vi "Competition.vi"() -> ()   [LabVIEW 2024]
uses:
  <vilib>/userDefined/High Color/IMAQdx.ctl
  System.Windows.Forms
  <vilib>/Instr/_visa.llb/VISA Set IO Buffer Mask.ctl
  <vilib>/Instr/_visa.llb/VISA Flush IO Buffer Mask.ctl
  e33ea129-5426-40bd-9da2-e127971607b1.vi
  <vilib>/Instr/_visa.llb/VISA Configure Serial Port (Instr).vi
  <vilib>/Python/Open Venv Python Session.vi
  <vilib>/Utility/file.llb/Read Delimited Spreadsheet (DBL).vi
  <vilib>/vision/driver/NI_Vision_Acquisition_Software.lvlib
panel:
  in  "RDDF":path=path "C:/Users/JungiHong/OneDrive/Hongik/HI-RACE/2026-01/ExperimentModules/GPSPathTracking/1_5_map/1_5_map hard.txt"
  out "WP_no.":i32=675
  out "Path_lat_arr":dbl[](array[numeric])=[250246.8301, 250246.6716, 250246.4873, 250246.296, 250246.122, 250245.9257, 250245.7732, 250245.5875, 250245.3989, 250245.2166, 250245.0276, 250244.8653, 250244.6749, 250244.5098, 250244.319, 250244.1293, 250243.9404, 250243.757, 250243.5653, 250243.3909, 250243.2171, 250243.0265, 250242.8469, 250242.6561, 250242.4779, 250242.2931, 250242.1112, 250241.9363, 250241.7611, 250241.5908]
  out "Path_long_arr":dbl[](array[numeric])=[3688223.612, 3688223.681, 3688223.731, 3688223.77, 3688223.796, 3688223.82, 3688223.842, 3688223.793, 3688223.791, 3688223.745, 3688223.702, 3688223.665, 3688223.63, 3688223.575, 3688223.538, 3688223.496, 3688223.445, 3688223.39, 3688223.345, 3688223.293, 3688223.242, 3688223.21, 3688223.151, 3688223.108, 3688223.058, 3688223.007, 3688222.954, 3688222.905, 3688222.836, 3688222.787]
  out "Path_Vel_arr":dbl[](array[numeric])=[126.3175841, 126.3175824, 126.3175804, 126.3175784, 126.3175765, 126.3175744, 126.3175727, 126.3175708, 126.3175687, 126.3175668, 126.3175648, 126.3175631, 126.317561, 126.3175593, 126.3175572, 126.3175552, 126.3175532, 126.3175512, 126.3175492, 126.3175473, 126.3175455, 126.3175434, 126.3175415, 126.3175395, 126.3175376, 126.3175356, 126.3175337, 126.3175318, 126.31753, 126.3175282]
  out "Path_Evt_arr":dbl[](array[numeric])=[33.30420584, 33.30420642, 33.30420683, 33.30420714, 33.30420733, 33.3042075, 33.30420766, 33.30420718, 33.30420712, 33.30420667, 33.30420623, 33.30420586, 33.3042055, 33.30420497, 33.30420459, 33.30420417, 33.30420367, 33.30420313, 33.30420267, 33.30420217, 33.30420167, 33.30420133, 33.30420076, 33.30420033, 33.30419983, 33.30419933, 33.30419882, 33.30419833, 33.30419768, 33.30419719]
  out "Evt":dbl
  in  "Map Refresh":bool
  out "X_lat_path_Full":dbl[](array[numeric])=[250204.6315, 250204.7847, 250204.9423, 250205.0812, 250205.2434, 250205.3871, 250205.5336, 250205.6795, 250205.8333, 250205.974, 250206.1254, 250206.2733, 250206.4155, 250206.5694, 250206.7606, 250206.9331, 250207.0915, 250207.2338, 250207.3801, 250207.5358, 250207.6911, 250207.8385, 250207.9859, 250208.1346, 250208.2889, 250208.4191, 250208.562, 250208.7088, 250208.8428, 250208.9854, 250209.1251, 250209.2579, 250209.3978, 250209.5384, 250209.6838, 250209.8317, 250209.9732, 250210.1069, 250210.2502, 250210.372, 250210.5044, 250210.6376, 250210.7611, 250210.9066, 250211.0503, 250211.1744, 250211.309, 250211.4462, 250211.5776, 250211.7104, 250211.8353, 250211.9552, 250212.0902, 250212.213, 250212.3298, 250212.4572, 250212.5757, 250212.6937, 250212.8209, 250212.9386, 250213.0558, 250213.1735, 250213.2937, 250213.4125, 250213.5502, 250213.6657, 250213.7946, 250213.9274, 250214.0472, 250214.1724, 250214.3017, 250214.4417, 250214.5753, 250214.7017, 250214.8378, 250214.9662, 250215.0894, 250215.2277, 250215.372, 250215.5023, 250215.6465, 250215.6465, 250215.7658, 250215.8914, 250216.017, 250216.142, 250216.2785, 250216.4267, 250216.5776, 250216.7312, 250216.8879, 250217.0506, 250217.2131, 250217.3799, 250217.5426, 250217.7046, 250217.8748, 250218.0423, 250218.2058, 250218.3739, 250218.5355, 250218.7031, 250218.8647, 250219.0346, 250219.1961, 250219.3482, 250219.5145, 250219.672, 250219.8212, 250219.9767, 250220.1301, 250220.2837, 250220.4332, 250220.5777, 250220.7226, 250220.8672, 250221.0139, 250221.1635, 250221.2913, 250221.4361, 250221.5854, 250221.7202, 250221.862, 250222.0043, 250222.1442, 250222.2947, 250222.4297, 250222.5803, 250222.7124, 250222.8553, 250222.9875, 250223.1252, 250223.2779, 250223.409, 250223.5472, 250223.6863, 250223.8257, 250223.9601, 250224.1026, 250224.2408, 250224.3821, 250224.528, 250224.675, 250224.8272, 250224.9781, 250225.124, 250225.2738, 250225.4183, 250225.5696, 250225.7148, 250225.8666, 250226.0158, 250226.1696, 250226.314, 250226.464, 250226.616, 250226.7669, 250226.8995, 250227.0551, 250227.2017, 250227.3491, 250227.4987, 250227.651, 250227.8032, 250227.9491, 250228.1012, 250228.2468, 250228.3977, 250228.5421, 250228.6906, 250228.8411, 250228.9881, 250229.1171, 250229.2733, 250229.4177, 250229.5665, 250229.7135, 250229.8553, 250229.9955, 250230.1399, 250230.2778, 250230.4184, 250230.5592, 250230.6982, 250230.8426, 250230.9741, 250231.1183, 250231.2583, 250231.3917, 250231.5316, 250231.664, 250231.809, 250231.9365, 250232.0794, 250232.2326, 250232.3781, 250232.5288, 250232.6849, 250232.849, 250233.0169, 250233.1898, 250233.3618, 250233.5347, 250233.7129, 250233.8854, 250234.0582, 250234.2271, 250234.392, 250234.5465, 250234.6882, 250234.8252, 250234.962, 250235.0951, 250235.2304, 250235.3491, 250235.4717, 250235.6036, 250235.7176, 250235.8287, 250235.9455, 250236.054, 250236.1492, 250236.2337, 250236.312, 250236.3794, 250236.4369, 250236.4842, 250236.5555, 250236.5952, 250236.6264, 250236.6586, 250236.6755, 250236.6895, 250236.6942, 250236.697, 250236.6851, 250236.6654, 250236.6292, 250236.5933, 250236.551, 250236.4843, 250236.4291, 250236.3642, 250236.3049, 250236.2381, 250236.1715, 250236.0948, 250236.0356, 250235.9406, 250235.8714, 250235.7898, 250235.7058, 250235.658, 250235.5758, 250235.4943, 250235.4193, 250235.3767, 250235.3402, 250235.2889, 250235.2668, 250235.2332, 250235.1891, 250235.1614, 250235.1565, 250235.1204, 250235.1167, 250235.133, 250235.1628, 250235.1974, 250235.2612, 250235.3531, 250235.4155, 250235.5356, 250235.6584, 250235.7924, 250235.9326, 250236.0835, 250236.1855, 250236.3061, 250236.46, 250236.5583, 250236.7204, 250236.8858, 250237.0619, 250237.2443, 250237.4126, 250237.579, 250237.7347, 250237.9052, 250238.0628, 250238.1948, 250238.3334, 250238.4969, 250238.6626, 250238.831, 250239.0118, 250239.1778, 250239.3373, 250239.5311, 250239.6876, 250239.8513, 250240.05, 250240.2334, 250240.4321, 250240.6256, 250240.816, 250240.9998, 250241.1899, 250241.3681, 250241.5524, 250241.7339, 250241.9189, 250242.1048, 250242.2826, 250242.4514, 250242.6353, 250242.8115, 250242.986, 250243.1671, 250243.3465, 250243.5187, 250243.6972, 250243.888, 250244.084, 250244.2833, 250244.4766, 250244.6711, 250244.8658, 250245.0556, 250245.2439, 250245.4299, 250245.6119, 250245.7785, 250245.9451, 250246.096, 250246.2496, 250246.3875, 250246.5144, 250246.631, 250246.7342, 250246.8204, 250246.907, 250247.0092, 250247.1016, 250247.193, 250247.2639, 250247.3441, 250247.421, 250247.4764, 250247.5347, 250247.5768, 250247.6199, 250247.652, 250247.665, 250247.6714, 250247.6666, 250247.6394, 250247.6096, 250247.5413, 250247.498, 250247.4546, 250247.3884, 250247.3334, 250247.2883, 250247.2288, 250247.1836, 250247.1639, 250247.1466, 250247.1079, 250247.1021, 250247.0827, 250247.0531, 250247.0114, 250247.0067, 250246.9862, 250246.9811, 250246.9938, 250247.0308, 250247.0702, 250247.135, 250247.2146, 250247.3014, 250247.4225, 250247.5588, 250247.6858, 250247.828, 250247.9565, 250248.126, 250248.2664, 250248.409, 250248.5611, 250248.7068, 250248.8531, 250249.0229, 250249.202, 250249.3857, 250249.5753, 250249.7637, 250249.959, 250250.1426, 250250.3367, 250250.5143, 250250.6887, 250250.882, 250251.0751, 250251.2683, 250251.4599, 250251.6407, 250251.8269, 250252.0222, 250252.215, 250252.3883, 250252.58, 250252.7757, 250252.9624, 250253.1529, 250253.3403, 250253.5294, 250253.7184, 250253.907, 250254.0796, 250254.2588, 250254.4147, 250254.5819, 250254.743, 250254.8895, 250255.0112, 250255.1568, 250255.2877, 250255.437, 250255.5889, 250255.7462, 250255.9147, 250256.0842, 250256.2597, 250256.4476, 250256.6251, 250256.814, 250257.0016, 250257.1907, 250257.383, 250257.5732, 250257.7644, 250257.9556, 250258.1438, 250258.3228, 250258.5095, 250258.6883, 250258.8678, 250259.0368, 250259.2086, 250259.3646, 250259.5205, 250259.6669, 250259.7981, 250259.9204, 250260.0341, 250260.1304, 250260.2154, 250260.2683, 250260.3212, 250260.3713, 250260.4074, 250260.4278, 250260.4483, 250260.4538, 250260.4584, 250260.4638, 250260.4531, 250260.4269, 250260.4025, 250260.3748, 250260.3569, 250260.3259, 250260.306, 250260.3019, 250260.2913, 250260.2964, 250260.3013, 250260.322, 250260.3442, 250260.3803, 250260.414, 250260.462, 250260.5251, 250260.6072, 250260.6942, 250260.7672, 250260.8711, 250260.9697, 250261.0724, 250261.1817, 250261.2963, 250261.3941, 250261.4821, 250261.569, 250261.6706, 250261.7652, 250261.857, 250261.9183, 250261.9427, 250261.9912, 250261.9961, 250262.0007, 250261.9756, 250261.9489, 250261.9099, 250261.8812, 250261.8445, 250261.7817, 250261.7129, 250261.6398, 250261.5329, 250261.4604, 250261.3434, 250261.24, 250261.1259, 250260.9928, 250260.8741, 250260.7678, 250260.6137, 250260.4623, 250260.2939, 250260.126, 250259.9411, 250259.7546, 250259.5669, 250259.4199, 250259.2239, 250259.0425, 250258.8499, 250258.6584, 250258.475, 250258.2939, 250258.1037, 250257.9137, 250257.7231, 250257.5553, 250257.3716, 250257.2069, 250257.0301, 250256.8666, 250256.6854, 250256.514, 250256.3482, 250256.1782, 250256.0288, 250255.8463, 250255.6842, 250255.5166, 250255.3463, 250255.1982, 250255.0421, 250254.892, 250254.7261, 250254.5713, 250254.4091, 250254.2573, 250254.0995, 250253.9355, 250253.7624, 250253.5867, 250253.3985, 250253.2139, 250253.0287, 250252.8354, 250252.6448, 250252.4492, 250252.2513, 250252.0571, 250251.8685, 250251.6866, 250251.5105, 250251.3443, 250251.1824, 250251.0309, 250250.8789, 250250.7367, 250250.5995, 250250.4539, 250250.3121, 250250.1719, 250250.0299, 250249.887, 250249.7463, 250249.6052, 250249.4649, 250249.331, 250249.1893, 250249.0528, 250248.9386, 250248.8243, 250248.7236, 250248.6306, 250248.529, 250248.4359, 250248.3517, 250248.2827, 250248.2037, 250248.1463, 250248.0957, 250248.0509, 250248.0219, 250248.0051, 250247.9945, 250247.9837, 250247.989, 250247.9941, 250247.9993, 250248.0044, 250248.0095, 250248.0145, 250248.0352, 250248.0557, 250248.0919, 250248.1148, 250248.1615, 250248.1868, 250248.2214, 250248.2728, 250248.3179, 250248.3416, 250248.3511, 250248.3839, 250248.4042, 250248.432, 250248.4459, 250248.4908, 250248.5037, 250248.5435, 250248.5875, 250248.6237, 250248.6436, 250248.6662, 250248.6992, 250248.705, 250248.7258, 250248.7267, 250248.7214, 250248.7308, 250248.744, 250248.7337, 250248.7226, 250248.6855, 250248.6674, 250248.5843, 250248.537, 250248.448, 250248.3765, 250248.2712, 250248.1941, 250248.1144, 250247.9992, 250247.891, 250247.7807, 250247.6307, 250247.5171, 250247.3602, 250247.1874, 250247.0166, 250246.8301, 250246.6716, 250246.4873, 250246.296, 250246.122, 250245.9257, 250245.7732, 250245.5875, 250245.3989, 250245.2166, 250245.0276, 250244.8653, 250244.6749, 250244.5098, 250244.319, 250244.1293, 250243.9404, 250243.757, 250243.5653, 250243.3909, 250243.2171, 250243.0265, 250242.8469, 250242.6561, 250242.4779, 250242.2931, 250242.1112, 250241.9363, 250241.7611, 250241.5908, 250241.4105, 250241.2326, 250241.0415, 250240.8823, 250240.7086, 250240.5237, 250240.3385, 250240.1546, 250239.9595, 250239.7651, 250239.5694, 250239.3713, 250239.1737, 250238.9795, 250238.7874, 250238.5977, 250238.4158, 250238.2247, 250238.0451, 250237.867, 250237.6942, 250237.5189, 250237.359, 250237.1898, 250237.0315, 250236.8728, 250236.7137, 250236.5718, 250236.437, 250236.2994, 250236.1879, 250236.0639, 250235.9389, 250235.83, 250235.7229, 250235.6297, 250235.5351, 250235.4494, 250235.3697, 250235.3065, 250235.2435, 250235.1994, 250235.1375, 250235.0894, 250235.041, 250235.0127, 250234.9717, 250234.9373, 250234.9195, 250234.8912, 250234.852, 250234.8256, 250234.8066, 250234.7894, 250234.7971, 250234.798, 250234.7875, 250234.8083, 250234.8039, 250234.8027, 250234.8079, 250234.813, 250234.8181, 250234.8119, 250234.8202, 250234.8152, 250234.8222, 250234.8216, 250234.7975, 250234.7903, 250234.7485, 250234.7087, 250234.6504, 250234.616, 250234.567, 250234.5014, 250234.4497, 250234.3789, 250234.3334, 250234.2602, 250234.1655, 250234.0706, 250233.9596, 250233.8482, 250233.6928, 250233.5374, 250233.4092, 250233.2698, 250233.1115, 250232.9573, 250232.785, 250232.598, 250232.4051, 250232.2295, 250232.0509, 250231.866, 250231.6857, 250231.4995, 250231.3134, 250231.1433, 250230.9457, 250230.7492, 250230.5768, 250230.3831, 250230.1894, 250229.9975, 250229.8111, 250229.6241, 250229.4384, 250229.2517, 250229.069, 250228.8781, 250228.6895, 250228.511, 250228.3291, 250228.1418, 250227.9599, 250227.7698, 250227.597, 250227.4079, 250227.2175, 250227.0293, 250226.8363, 250226.6397, 250226.4445, 250226.4445, 250226.3195, 250226.1946, 250226.0696, 250225.9221, 250225.7742, 250225.6168, 250225.47, 250225.3233, 250225.1765, 250225.0287, 250224.8822, 250224.7443, 250224.5996, 250224.4528, 250224.301, 250224.1558, 250224.0269, 250223.8866, 250223.7351, 250223.5855, 250223.4444, 250223.2886, 250223.148, 250223.0104, 250222.8695, 250222.7295, 250222.5838, 250222.4554, 250222.316, 250222.1912, 250222.056, 250221.9297, 250221.7922, 250221.6642, 250221.5466, 250221.3995, 250221.2768, 250221.1432, 250221.0095, 250220.8891, 250220.7597, 250220.6502, 250220.5287, 250220.4116, 250220.2851, 250220.1647, 250220.0444, 250219.9261, 250219.7966, 250219.6741, 250219.5628, 250219.4354, 250219.3182, 250219.1887, 250219.0582, 250218.9251, 250218.8036, 250218.679, 250218.5495, 250218.4169, 250218.2866, 250218.1513, 250218.0199, 250217.8896, 250217.7568, 250217.6185, 250217.4845, 250217.3551, 250217.2166, 250217.0853, 250216.9453, 250216.8055, 250216.6585, 250216.5131, 250216.3689, 250216.2118, 250216.0655, 250215.9129, 250215.7606, 250215.6071, 250215.4505, 250215.2942, 250215.1411, 250214.9841, 250214.842, 250214.6871, 250214.5483, 250214.3987, 250214.2557, 250214.1195, 250213.9747, 250213.8377, 250213.7044, 250213.5703, 250213.4445, 250213.3184, 250213.183, 250213.0559, 250212.9317, 250212.8112, 250212.6789, 250212.5512, 250212.4267, 250212.2918, 250212.1645, 250212.0429, 250211.9046, 250211.769, 250211.6308, 250211.492, 250211.3609, 250211.2259, 250211.0952, 250210.9578, 250210.8141, 250210.6818, 250210.5388, 250210.4096, 250210.2669, 250210.1265, 250209.986, 250209.8443, 250209.696, 250209.5582, 250209.4275, 250209.2882, 250209.1319, 250209.0284]
  out "vel. path":dbl[](array[numeric])=[126.317125, 126.3171267, 126.3171284, 126.3171299, 126.3171317, 126.3171333, 126.3171349, 126.3171365, 126.3171382, 126.3171397, 126.3171414, 126.317143, 126.3171446, 126.3171463, 126.3171483, 126.3171502, 126.317152, 126.3171535, 126.3171551, 126.3171568, 126.3171585, 126.3171601, 126.3171618, 126.3171634, 126.3171651, 126.3171665, 126.3171681, 126.3171697, 126.3171712, 126.3171728, 126.3171743, 126.3171758, 126.3171773, 126.3171788, 126.3171804, 126.3171821, 126.3171836, 126.3171851, 126.3171867, 126.317188, 126.3171895, 126.317191, 126.3171923, 126.3171939, 126.3171955, 126.3171969, 126.3171984, 126.3171999, 126.3172013, 126.3172028, 126.3172042, 126.3172055, 126.317207, 126.3172083, 126.3172096, 126.3172111, 126.3172124, 126.3172137, 126.3172151, 126.3172164, 126.3172177, 126.317219, 126.3172203, 126.3172217, 126.3172232, 126.3172245, 126.3172259, 126.3172273, 126.3172287, 126.3172301, 126.3172315, 126.317233, 126.3172345, 126.3172359, 126.3172374, 126.3172388, 126.3172402, 126.3172417, 126.3172433, 126.3172447, 126.3172463, 126.3172463, 126.3172476, 126.317249, 126.3172504, 126.3172518, 126.3172533, 126.3172549, 126.3172566, 126.3172583, 126.31726, 126.3172618, 126.3172635, 126.3172654, 126.3172671, 126.3172689, 126.3172708, 126.3172726, 126.3172744, 126.3172762, 126.317278, 126.3172798, 126.3172816, 126.3172834, 126.3172852, 126.3172868, 126.3172886, 126.3172904, 126.317292, 126.3172937, 126.3172954, 126.3172971, 126.3172987, 126.3173003, 126.3173019, 126.3173035, 126.3173051, 126.3173067, 126.3173081, 126.3173097, 126.3173114, 126.3173129, 126.3173144, 126.317316, 126.3173175, 126.3173192, 126.3173207, 126.3173223, 126.3173238, 126.3173253, 126.3173268, 126.3173283, 126.31733, 126.3173314, 126.317333, 126.3173345, 126.317336, 126.3173375, 126.3173391, 126.3173406, 126.3173421, 126.3173437, 126.3173454, 126.317347, 126.3173487, 126.3173503, 126.3173519, 126.3173535, 126.3173552, 126.3173568, 126.3173584, 126.3173601, 126.3173617, 126.3173633, 126.317365, 126.3173666, 126.3173683, 126.3173698, 126.3173715, 126.3173731, 126.3173747, 126.3173763, 126.317378, 126.3173797, 126.3173813, 126.3173829, 126.3173845, 126.3173862, 126.3173878, 126.3173894, 126.3173911, 126.3173927, 126.3173941, 126.3173958, 126.3173974, 126.317399, 126.3174006, 126.3174022, 126.3174037, 126.3174053, 126.3174068, 126.3174084, 126.3174099, 126.3174115, 126.3174131, 126.3174145, 126.3174161, 126.3174176, 126.3174191, 126.3174206, 126.3174221, 126.3174237, 126.3174251, 126.3174267, 126.3174284, 126.31743, 126.3174316, 126.3174333, 126.3174351, 126.3174369, 126.3174388, 126.3174407, 126.3174426, 126.3174445, 126.3174464, 126.3174483, 126.3174501, 126.3174519, 126.3174536, 126.3174552, 126.3174567, 126.3174582, 126.3174596, 126.3174611, 126.3174624, 126.3174638, 126.3174653, 126.3174665, 126.3174678, 126.3174691, 126.3174703, 126.3174713, 126.3174723, 126.3174732, 126.317474, 126.3174746, 126.3174752, 126.317476, 126.3174765, 126.3174769, 126.3174773, 126.3174775, 126.3174777, 126.3174778, 126.3174779, 126.3174778, 126.3174777, 126.3174773, 126.317477, 126.3174766, 126.3174759, 126.3174754, 126.3174748, 126.3174742, 126.3174735, 126.3174728, 126.3174721, 126.3174715, 126.3174705, 126.3174698, 126.317469, 126.3174681, 126.3174677, 126.3174668, 126.317466, 126.3174653, 126.3174648, 126.3174645, 126.317464, 126.3174638, 126.3174635, 126.3174631, 126.3174628, 126.3174628, 126.3174625, 126.3174625, 126.3174627, 126.3174631, 126.3174635, 126.3174643, 126.3174653, 126.317466, 126.3174673, 126.3174687, 126.3174702, 126.3174717, 126.3174734, 126.3174745, 126.3174758, 126.3174775, 126.31747849999999, 126.3174803, 126.3174821, 126.317484, 126.317486, 126.3174878, 126.3174896, 126.3174913, 126.3174932, 126.3174949, 126.3174963, 126.3174978, 126.3174996, 126.3175014, 126.3175032, 126.3175052, 126.317507, 126.3175087, 126.3175108, 126.3175125, 126.3175142, 126.3175164, 126.3175183, 126.3175205, 126.3175225, 126.3175246, 126.3175265, 126.3175286, 126.3175305, 126.3175324, 126.3175344, 126.3175363, 126.3175383, 126.3175402, 126.317542, 126.3175439, 126.3175458, 126.3175477, 126.3175496, 126.3175515, 126.3175533, 126.3175552, 126.3175573, 126.3175594, 126.3175615, 126.3175636, 126.3175657, 126.3175678, 126.3175698, 126.3175719, 126.3175739, 126.3175759, 126.3175777, 126.3175795, 126.3175811, 126.3175828, 126.3175843, 126.3175857, 126.317587, 126.3175882, 126.3175892, 126.3175901, 126.3175913, 126.3175923, 126.3175933, 126.3175942, 126.3175951, 126.3175959, 126.3175966, 126.3175973, 126.3175978, 126.3175983, 126.3175987, 126.3175989, 126.317599, 126.317599, 126.3175988, 126.3175985, 126.3175978, 126.3175974, 126.317597, 126.3175963, 126.3175958, 126.3175954, 126.3175948, 126.3175943, 126.3175942, 126.317594, 126.3175937, 126.3175937, 126.3175935, 126.3175932, 126.3175928, 126.3175928, 126.3175927, 126.3175927, 126.3175929, 126.3175933, 126.3175938, 126.3175945, 126.3175954, 126.3175964, 126.3175977, 126.3175992, 126.3176006, 126.3176022, 126.3176036, 126.3176055, 126.317607, 126.3176086, 126.3176102, 126.3176118, 126.3176134, 126.3176152, 126.3176172, 126.3176192, 126.3176212, 126.3176233, 126.3176254, 126.3176274, 126.3176294, 126.3176314, 126.3176333, 126.3176353, 126.3176374, 126.3176395, 126.3176416, 126.3176435, 126.3176455, 126.3176476, 126.3176497, 126.3176515, 126.3176536, 126.3176557, 126.3176577, 126.3176597, 126.3176617, 126.3176637, 126.3176657, 126.3176677, 126.3176696, 126.3176715, 126.3176731, 126.3176749, 126.3176766, 126.3176781, 126.3176794, 126.3176809, 126.3176823, 126.3176838, 126.3176854, 126.3176871, 126.3176889, 126.3176906, 126.3176925, 126.3176945, 126.3176964, 126.3176984, 126.3177004, 126.3177024, 126.3177044, 126.3177065, 126.3177085, 126.3177106, 126.3177126, 126.3177145, 126.3177164, 126.3177183, 126.3177202, 126.317722, 126.3177238, 126.3177255, 126.3177271, 126.3177287, 126.31773, 126.3177313, 126.3177325, 126.3177335, 126.3177343, 126.3177348, 126.3177353, 126.3177358, 126.3177362, 126.3177363, 126.3177365, 126.3177365, 126.3177365, 126.3177365, 126.3177363, 126.317736, 126.3177357, 126.3177353, 126.3177351, 126.3177347, 126.3177344, 126.3177343, 126.3177342, 126.3177342, 126.3177342, 126.3177343, 126.3177345, 126.3177349, 126.3177352, 126.3177356, 126.3177362, 126.3177371, 126.317738, 126.3177387, 126.3177398, 126.3177408, 126.3177418, 126.317743, 126.3177441, 126.3177452, 126.317746, 126.3177469, 126.317748, 126.3177489, 126.3177499, 126.3177505, 126.3177507, 126.3177512, 126.3177512, 126.3177512, 126.3177508, 126.3177505, 126.31775, 126.3177497, 126.3177492, 126.3177485, 126.3177477, 126.3177469, 126.3177457, 126.3177449, 126.3177436, 126.3177424, 126.3177412, 126.3177397, 126.3177384, 126.3177372, 126.3177355, 126.3177339, 126.317732, 126.3177302, 126.3177282, 126.3177262, 126.3177242, 126.3177226, 126.3177205, 126.3177186, 126.3177165, 126.3177145, 126.3177125, 126.3177106, 126.3177085, 126.3177065, 126.3177045, 126.3177027, 126.3177007, 126.317699, 126.3176971, 126.3176954, 126.3176934, 126.3176916, 126.3176899, 126.3176881, 126.3176865, 126.3176845, 126.3176828, 126.3176811, 126.3176793, 126.3176777, 126.317676, 126.3176745, 126.3176727, 126.3176711, 126.3176694, 126.3176678, 126.3176661, 126.3176644, 126.3176626, 126.3176607, 126.3176587, 126.3176567, 126.3176548, 126.3176527, 126.3176507, 126.3176486, 126.3176464, 126.3176444, 126.3176423, 126.3176403, 126.3176384, 126.3176366, 126.3176349, 126.3176332, 126.3176315, 126.31763, 126.3176285, 126.3176269, 126.3176253, 126.3176238, 126.3176222, 126.3176206, 126.3176191, 126.3176175, 126.317616, 126.3176145, 126.3176129, 126.3176114, 126.3176102, 126.3176089, 126.3176078, 126.3176067, 126.3176056, 126.3176045, 126.3176036, 126.3176028, 126.3176019, 126.3176012, 126.3176006, 126.3176001, 126.3175997, 126.3175995, 126.3175993, 126.3175992, 126.3175992, 126.3175992, 126.3175992, 126.3175992, 126.3175992, 126.3175992, 126.3175993, 126.3175995, 126.3175998, 126.3176, 126.3176005, 126.3176007, 126.317601, 126.3176015, 126.3176019, 126.3176022, 126.3176022, 126.3176025, 126.3176027, 126.3176029, 126.317603, 126.3176034, 126.3176035, 126.3176039, 126.3176043, 126.3176047, 126.3176048, 126.317605, 126.3176053, 126.3176053, 126.3176055, 126.3176055, 126.3176054, 126.3176054, 126.3176055, 126.3176053, 126.3176052, 126.3176047, 126.3176045, 126.3176035, 126.317603, 126.317602, 126.3176012, 126.3176, 126.3175991, 126.3175982, 126.3175969, 126.3175957, 126.3175945, 126.3175929, 126.3175916, 126.3175899, 126.317588, 126.3175862, 126.3175841, 126.3175824, 126.3175804, 126.3175784, 126.3175765, 126.3175744, 126.3175727, 126.3175708, 126.3175687, 126.3175668, 126.3175648, 126.3175631, 126.317561, 126.3175593, 126.3175572, 126.3175552, 126.3175532, 126.3175512, 126.3175492, 126.3175473, 126.3175455, 126.3175434, 126.3175415, 126.3175395, 126.3175376, 126.3175356, 126.3175337, 126.3175318, 126.31753, 126.3175282, 126.3175262, 126.3175243, 126.3175223, 126.3175206, 126.3175188, 126.3175168, 126.3175148, 126.3175129, 126.3175108, 126.3175087, 126.3175066, 126.3175045, 126.3175024, 126.3175003, 126.3174982, 126.3174961, 126.3174942, 126.3174921, 126.3174902, 126.3174882, 126.3174863, 126.3174844, 126.3174827, 126.3174809, 126.3174791, 126.3174774, 126.3174756, 126.3174741, 126.3174726, 126.3174711, 126.3174698, 126.3174685, 126.3174671, 126.3174659, 126.3174647, 126.3174636, 126.3174626, 126.3174616, 126.3174607, 126.31746, 126.3174592, 126.3174587, 126.317458, 126.3174574, 126.3174568, 126.3174565, 126.317456, 126.3174556, 126.3174553, 126.317455, 126.3174545, 126.3174542, 126.3174539, 126.3174537, 126.3174537, 126.3174537, 126.3174535, 126.3174537, 126.3174536, 126.3174535, 126.3174535, 126.3174535, 126.3174535, 126.3174534, 126.3174534, 126.3174533, 126.3174533, 126.3174533, 126.317453, 126.3174528, 126.3174523, 126.3174519, 126.3174512, 126.3174508, 126.3174502, 126.3174494, 126.3174488, 126.317448, 126.3174475, 126.3174467, 126.3174456, 126.3174445, 126.3174433, 126.3174421, 126.3174404, 126.3174387, 126.3174373, 126.3174358, 126.317434, 126.3174324, 126.3174305, 126.3174285, 126.3174264, 126.3174245, 126.3174226, 126.3174206, 126.3174187, 126.3174167, 126.3174147, 126.3174128, 126.3174107, 126.3174086, 126.3174068, 126.3174047, 126.3174026, 126.3174006, 126.3173986, 126.3173966, 126.3173946, 126.3173926, 126.3173907, 126.3173887, 126.3173867, 126.3173848, 126.3173828, 126.3173808, 126.3173789, 126.3173769, 126.317375, 126.317373, 126.317371, 126.317369, 126.3173669, 126.31736480000001, 126.3173627, 126.3173627, 126.3173614, 126.31736, 126.3173587, 126.3173571, 126.3173554, 126.3173537, 126.3173521, 126.3173505, 126.3173489, 126.3173473, 126.3173457, 126.3173441, 126.3173426, 126.3173409, 126.3173393, 126.3173377, 126.3173363, 126.3173347, 126.3173331, 126.3173314, 126.3173299, 126.3173282, 126.3173266, 126.3173251, 126.3173235, 126.317322, 126.3173204, 126.317319, 126.3173175, 126.3173161, 126.3173146, 126.3173132, 126.3173117, 126.3173103, 126.3173089, 126.3173073, 126.317306, 126.3173045, 126.317303, 126.3173017, 126.3173003, 126.317299, 126.3172977, 126.3172964, 126.317295, 126.3172937, 126.3172923, 126.317291, 126.3172896, 126.3172882, 126.317287, 126.3172856, 126.3172843, 126.3172829, 126.3172814, 126.31728, 126.3172786, 126.3172772, 126.3172758, 126.3172743, 126.3172729, 126.3172714, 126.31727, 126.3172685, 126.317267, 126.3172655, 126.317264, 126.3172626, 126.3172611, 126.3172596, 126.3172581, 126.3172566, 126.317255, 126.3172534, 126.3172518, 126.3172501, 126.3172485, 126.3172468, 126.3172451, 126.3172434, 126.3172417, 126.31724, 126.3172383, 126.3172366, 126.3172351, 126.3172334, 126.3172318, 126.3172302, 126.3172286, 126.3172271, 126.3172255, 126.317224, 126.3172225, 126.3172211, 126.3172197, 126.3172183, 126.3172168, 126.3172154, 126.317214, 126.3172127, 126.3172112, 126.3172098, 126.3172084, 126.3172069, 126.3172055, 126.3172042, 126.3172027, 126.3172012, 126.3171997, 126.3171981, 126.3171967, 126.3171952, 126.3171937, 126.3171922, 126.3171907, 126.3171892, 126.3171876, 126.3171862, 126.3171846, 126.3171831, 126.3171815, 126.31718, 126.3171783, 126.3171768, 126.3171754, 126.3171739, 126.3171721, 126.317171]
  out "Y_long_path_Full":dbl[](array[numeric])=[3688246.636, 3688246.509, 3688246.386, 3688246.252, 3688246.131, 3688245.999, 3688245.863, 3688245.725, 3688245.593, 3688245.45, 3688245.315, 3688245.179, 3688245.039, 3688244.911, 3688244.843, 3688244.735, 3688244.608, 3688244.485, 3688244.347, 3688244.225, 3688244.098, 3688243.962, 3688243.826, 3688243.702, 3688243.576, 3688243.428, 3688243.289, 3688243.152, 3688243.019, 3688242.881, 3688242.758, 3688242.611, 3688242.466, 3688242.324, 3688242.184, 3688242.046, 3688241.912, 3688241.761, 3688241.621, 3688241.464, 3688241.317, 3688241.168, 3688241.016, 3688240.878, 3688240.743, 3688240.587, 3688240.445, 3688240.302, 3688240.154, 3688240.007, 3688239.85, 3688239.697, 3688239.549, 3688239.391, 3688239.229, 3688239.078, 3688238.919, 3688238.759, 3688238.606, 3688238.449, 3688238.288, 3688238.132, 3688237.972, 3688237.812, 3688237.667, 3688237.509, 3688237.359, 3688237.212, 3688237.056, 3688236.903, 3688236.761, 3688236.618, 3688236.472, 3688236.318, 3688236.18, 3688236.04, 3688235.882, 3688235.736, 3688235.602, 3688235.455, 3688235.317, 3688235.317, 3688235.161, 3688235.009, 3688234.859, 3688234.707, 3688234.563, 3688234.431, 3688234.301, 3688234.177, 3688234.058, 3688233.945, 3688233.832, 3688233.726, 3688233.616, 3688233.504, 3688233.406, 3688233.302, 3688233.192, 3688233.09, 3688232.98, 3688232.875, 3688232.767, 3688232.663, 3688232.554, 3688232.429, 3688232.322, 3688232.207, 3688232.075, 3688231.951, 3688231.826, 3688231.702, 3688231.575, 3688231.444, 3688231.311, 3688231.182, 3688231.047, 3688230.919, 3688230.774, 3688230.641, 3688230.511, 3688230.367, 3688230.231, 3688230.094, 3688229.957, 3688229.829, 3688229.683, 3688229.557, 3688229.413, 3688229.278, 3688229.132, 3688228.991, 3688228.865, 3688228.717, 3688228.577, 3688228.436, 3688228.296, 3688228.16, 3688228.023, 3688227.884, 3688227.749, 3688227.618, 3688227.486, 3688227.365, 3688227.239, 3688227.103, 3688226.975, 3688226.839, 3688226.711, 3688226.574, 3688226.45, 3688226.318, 3688226.199, 3688226.063, 3688225.934, 3688225.812, 3688225.684, 3688225.54, 3688225.421, 3688225.29, 3688225.156, 3688225.028, 3688224.9, 3688224.772, 3688224.642, 3688224.516, 3688224.383, 3688224.257, 3688224.124, 3688223.994, 3688223.865, 3688223.735, 3688223.59, 3688223.474, 3688223.338, 3688223.207, 3688223.074, 3688222.936, 3688222.795, 3688222.659, 3688222.518, 3688222.382, 3688222.244, 3688222.105, 3688221.97, 3688221.825, 3688221.694, 3688221.554, 3688221.407, 3688221.266, 3688221.121, 3688220.986, 3688220.837, 3688220.7, 3688220.579, 3688220.446, 3688220.321, 3688220.2, 3688220.09, 3688219.984, 3688219.886, 3688219.791, 3688219.695, 3688219.609, 3688219.511, 3688219.412, 3688219.312, 3688219.202, 3688219.08, 3688218.943, 3688218.802, 3688218.658, 3688218.514, 3688218.373, 3688218.215, 3688218.06, 3688217.916, 3688217.752, 3688217.592, 3688217.434, 3688217.271, 3688217.096, 3688216.918, 3688216.738, 3688216.555, 3688216.364, 3688216.175, 3688215.99, 3688215.797, 3688215.603, 3688215.408, 3688215.212, 3688215.018, 3688214.825, 3688214.629, 3688214.435, 3688214.238, 3688214.045, 3688213.854, 3688213.659, 3688213.473, 3688213.282, 3688213.096, 3688212.911, 3688212.732, 3688212.553, 3688212.373, 3688212.187, 3688212.026, 3688211.845, 3688211.666, 3688211.498, 3688211.307, 3688211.137, 3688210.957, 3688210.774, 3688210.583, 3688210.455, 3688210.27, 3688210.079, 3688209.89, 3688209.707, 3688209.511, 3688209.32, 3688209.133, 3688208.944, 3688208.778, 3688208.603, 3688208.425, 3688208.24, 3688208.069, 3688207.923, 3688207.776, 3688207.638, 3688207.505, 3688207.376, 3688207.261, 3688207.163, 3688207.105, 3688206.993, 3688206.89, 3688206.843, 3688206.777, 3688206.715, 3688206.655, 3688206.559, 3688206.461, 3688206.366, 3688206.273, 3688206.184, 3688206.113, 3688205.99, 3688205.895, 3688205.827, 3688205.775, 3688205.706, 3688205.658, 3688205.603, 3688205.616, 3688205.607, 3688205.608, 3688205.602, 3688205.579, 3688205.574, 3688205.595, 3688205.626, 3688205.67, 3688205.702, 3688205.765, 3688205.832, 3688205.892, 3688205.924, 3688205.975, 3688206.044, 3688206.125, 3688206.183, 3688206.249, 3688206.333, 3688206.409, 3688206.446, 3688206.526, 3688206.566, 3688206.595, 3688206.609, 3688206.603, 3688206.58, 3688206.556, 3688206.533, 3688206.491, 3688206.441, 3688206.381, 3688206.31, 3688206.213, 3688206.118, 3688205.996, 3688205.876, 3688205.735, 3688205.585, 3688205.428, 3688205.261, 3688205.087, 3688204.913, 3688204.745, 3688204.572, 3688204.399, 3688204.217, 3688204.041, 3688203.86, 3688203.671, 3688203.482, 3688203.291, 3688203.097, 3688202.903, 3688202.706, 3688202.51, 3688202.313, 3688202.121, 3688201.928, 3688201.742, 3688201.55, 3688201.357, 3688201.175, 3688201.009, 3688200.831, 3688200.66, 3688200.469, 3688200.293, 3688200.102, 3688199.927, 3688199.75, 3688199.553, 3688199.364, 3688199.207, 3688199.015, 3688198.819, 3688198.62, 3688198.43, 3688198.239, 3688198.051, 3688197.866, 3688197.706, 3688197.53, 3688197.389, 3688197.254, 3688197.113, 3688197.004, 3688196.877, 3688196.777, 3688196.671, 3688196.564, 3688196.467, 3688196.356, 3688196.256, 3688196.178, 3688196.107, 3688196.03, 3688195.977, 3688195.933, 3688195.904, 3688195.84, 3688195.809, 3688195.77, 3688195.714, 3688195.686, 3688195.663, 3688195.635, 3688195.597, 3688195.593, 3688195.569, 3688195.582, 3688195.578, 3688195.592, 3688195.622, 3688195.638, 3688195.688, 3688195.721, 3688195.771, 3688195.83, 3688195.888, 3688195.924, 3688196.013, 3688196.097, 3688196.199, 3688196.297, 3688196.407, 3688196.538, 3688196.689, 3688196.822, 3688196.969, 3688197.098, 3688197.223, 3688197.336, 3688197.437, 3688197.537, 3688197.627, 3688197.689, 3688197.772, 3688197.835, 3688197.898, 3688197.962, 3688198.006, 3688198.066, 3688198.118, 3688198.16, 3688198.22, 3688198.3, 3688198.363, 3688198.445, 3688198.523, 3688198.622, 3688198.722, 3688198.834, 3688198.951, 3688199.084, 3688199.233, 3688199.389, 3688199.552, 3688199.724, 3688199.899, 3688200.09, 3688200.276, 3688200.466, 3688200.659, 3688200.855, 3688201.049, 3688201.243, 3688201.442, 3688201.641, 3688201.837, 3688202.031, 3688202.224, 3688202.419, 3688202.615, 3688202.809, 3688203.003, 3688203.2, 3688203.398, 3688203.596, 3688203.795, 3688203.99, 3688204.187, 3688204.382, 3688204.576, 3688204.768, 3688204.955, 3688205.134, 3688205.302, 3688205.48, 3688205.649, 3688205.819, 3688205.987, 3688206.153, 3688206.315, 3688206.475, 3688206.647, 3688206.821, 3688206.984, 3688207.155, 3688207.331, 3688207.516, 3688207.707, 3688207.883, 3688208.081, 3688208.28, 3688208.475, 3688208.668, 3688208.858, 3688209.044, 3688209.226, 3688209.406, 3688209.585, 3688209.736, 3688209.892, 3688210.061, 3688210.21, 3688210.376, 3688210.537, 3688210.657, 3688210.774, 3688210.911, 3688211.029, 3688211.149, 3688211.236, 3688211.32, 3688211.383, 3688211.44, 3688211.445, 3688211.43, 3688211.417, 3688211.403, 3688211.371, 3688211.339, 3688211.288, 3688211.266, 3688211.231, 3688211.192, 3688211.159, 3688211.09, 3688211.04, 3688210.987, 3688210.902, 3688210.837, 3688210.775, 3688210.694, 3688210.621, 3688210.559, 3688210.478, 3688210.405, 3688210.295, 3688210.196, 3688210.103, 3688209.986, 3688209.897, 3688209.77, 3688209.673, 3688209.572, 3688209.462, 3688209.359, 3688209.244, 3688209.133, 3688209.036, 3688208.949, 3688208.891, 3688208.817, 3688208.749, 3688208.713, 3688208.664, 3688208.65, 3688208.66, 3688208.683, 3688208.737, 3688208.812, 3688208.9, 3688209.001, 3688209.113, 3688209.24, 3688209.367, 3688209.505, 3688209.64, 3688209.773, 3688209.904, 3688210.04, 3688210.178, 3688210.315, 3688210.453, 3688210.59, 3688210.727, 3688210.871, 3688211.008, 3688211.148, 3688211.311, 3688211.471, 3688211.642, 3688211.815, 3688211.983, 3688212.159, 3688212.339, 3688212.521, 3688212.701, 3688212.891, 3688213.083, 3688213.276, 3688213.469, 3688213.666, 3688213.862, 3688214.057, 3688214.255, 3688214.453, 3688214.653, 3688214.853, 3688215.051, 3688215.25, 3688215.444, 3688215.641, 3688215.834, 3688216.03, 3688216.22, 3688216.415, 3688216.609, 3688216.798, 3688216.975, 3688217.146, 3688217.341, 3688217.523, 3688217.718, 3688217.904, 3688218.088, 3688218.264, 3688218.452, 3688218.624, 3688218.803, 3688218.991, 3688219.18, 3688219.365, 3688219.554, 3688219.748, 3688219.937, 3688220.115, 3688220.312, 3688220.462, 3688220.658, 3688220.856, 3688221.033, 3688221.218, 3688221.387, 3688221.55, 3688221.723, 3688221.888, 3688222.066, 3688222.206, 3688222.378, 3688222.54, 3688222.688, 3688222.84, 3688222.985, 3688223.105, 3688223.246, 3688223.363, 3688223.459, 3688223.551, 3688223.612, 3688223.681, 3688223.731, 3688223.77, 3688223.796, 3688223.82, 3688223.842, 3688223.793, 3688223.791, 3688223.745, 3688223.702, 3688223.665, 3688223.63, 3688223.575, 3688223.538, 3688223.496, 3688223.445, 3688223.39, 3688223.345, 3688223.293, 3688223.242, 3688223.21, 3688223.151, 3688223.108, 3688223.058, 3688223.007, 3688222.954, 3688222.905, 3688222.836, 3688222.787, 3688222.74, 3688222.683, 3688222.638, 3688222.586, 3688222.511, 3688222.478, 3688222.412, 3688222.359, 3688222.34, 3688222.314, 3688222.3, 3688222.305, 3688222.31, 3688222.337, 3688222.376, 3688222.424, 3688222.483, 3688222.527, 3688222.608, 3688222.689, 3688222.783, 3688222.873, 3688222.992, 3688223.093, 3688223.213, 3688223.334, 3688223.454, 3688223.591, 3688223.737, 3688223.876, 3688224.034, 3688224.188, 3688224.344, 3688224.508, 3688224.673, 3688224.847, 3688225.02, 3688225.2, 3688225.381, 3688225.567, 3688225.754, 3688225.947, 3688226.135, 3688226.326, 3688226.518, 3688226.714, 3688226.903, 3688227.091, 3688227.284, 3688227.478, 3688227.672, 3688227.866, 3688228.052, 3688228.244, 3688228.437, 3688228.601, 3688228.797, 3688228.994, 3688229.189, 3688229.387, 3688229.587, 3688229.785, 3688229.985, 3688230.183, 3688230.38, 3688230.566, 3688230.748, 3688230.94, 3688231.128, 3688231.318, 3688231.504, 3688231.693, 3688231.866, 3688232.053, 3688232.23, 3688232.388, 3688232.573, 3688232.725, 3688232.88, 3688233.054, 3688233.218, 3688233.39, 3688233.528, 3688233.686, 3688233.804, 3688233.914, 3688234.006, 3688234.079, 3688234.157, 3688234.233, 3688234.306, 3688234.361, 3688234.397, 3688234.42, 3688234.426, 3688234.413, 3688234.415, 3688234.412, 3688234.395, 3688234.411, 3688234.397, 3688234.384, 3688234.363, 3688234.325, 3688234.303, 3688234.255, 3688234.209, 3688234.17, 3688234.122, 3688234.08, 3688234.02, 3688233.976, 3688233.93, 3688233.866, 3688233.809, 3688233.757, 3688233.697, 3688233.665, 3688233.601, 3688233.564, 3688233.533, 3688233.503, 3688233.455, 3688233.435, 3688233.422, 3688233.422, 3688233.413, 3688233.405, 3688233.397, 3688233.525, 3688233.659, 3688233.778, 3688233.911, 3688234.043, 3688234.174, 3688234.307, 3688234.435, 3688234.569, 3688234.705, 3688234.84, 3688234.961, 3688235.097, 3688235.227, 3688235.365, 3688235.493, 3688235.623, 3688235.758, 3688235.877, 3688236.014, 3688236.159, 3688236.295, 3688236.435, 3688236.571, 3688236.724, 3688236.867, 3688237.018, 3688237.158, 3688237.308, 3688237.453, 3688237.606, 3688237.764, 3688237.899, 3688238.054, 3688238.201, 3688238.349, 3688238.502, 3688238.644, 3688238.795, 3688238.953, 3688239.112, 3688239.259, 3688239.41, 3688239.562, 3688239.702, 3688239.853, 3688240.006, 3688240.166, 3688240.313, 3688240.473, 3688240.61, 3688240.762, 3688240.907, 3688241.061, 3688241.213, 3688241.362, 3688241.508, 3688241.659, 3688241.804, 3688241.946, 3688242.094, 3688242.243, 3688242.387, 3688242.527, 3688242.67, 3688242.808, 3688242.951, 3688243.091, 3688243.229, 3688243.354, 3688243.482, 3688243.612, 3688243.732, 3688243.857, 3688243.981, 3688244.094, 3688244.219, 3688244.343, 3688244.466, 3688244.587, 3688244.708, 3688244.84, 3688244.965, 3688245.103, 3688245.229, 3688245.362, 3688245.503, 3688245.64, 3688245.78, 3688245.922, 3688246.064, 3688246.214, 3688246.361, 3688246.508, 3688246.655, 3688246.809, 3688246.962, 3688247.108, 3688247.256, 3688247.407, 3688247.548, 3688247.695, 3688247.846, 3688247.99, 3688248.13, 3688248.271, 3688248.412, 3688248.553, 3688248.699, 3688248.848, 3688248.992, 3688249.128, 3688249.276, 3688249.41, 3688249.556, 3688249.69, 3688249.832, 3688249.967, 3688250.104, 3688250.232, 3688250.375, 3688250.521, 3688250.658, 3688250.777, 3688250.901]
  out "Evt.Arr":dbl[](array[numeric])=[33.3044035, 33.3044024, 33.30440132, 33.30440015, 33.3043991, 33.30439794, 33.30439675, 33.30439554, 33.30439439, 33.30439313, 33.30439195, 33.30439076, 33.30438953, 33.30438841, 33.30438784, 33.30438692, 33.3043858, 33.30438473, 33.30438352, 33.30438245, 33.30438134, 33.30438015, 33.30437896, 33.30437788, 33.30437678, 33.30437548, 33.30437425, 33.30437306, 33.30437189, 33.30437068, 33.3043696, 33.30436831, 33.30436703, 33.30436578, 33.30436456, 33.30436336, 33.30436217, 33.30436085, 33.30435962, 33.30435823, 33.30435694, 33.30435563, 33.30435428, 33.30435308, 33.30435189, 33.30435052, 33.30434926, 33.30434801, 33.30434672, 33.30434541, 33.30434403, 33.30434268, 33.30434137, 33.30433998, 33.30433855, 33.30433722, 33.30433581, 33.3043344, 33.30433306, 33.30433166, 33.30433024, 33.30432886, 33.30432745, 33.30432603, 33.30432476, 33.30432336, 33.30432204, 33.30432075, 33.30431937, 33.30431801, 33.30431677, 33.30431551, 33.30431422, 33.30431287, 33.30431166, 33.30431043, 33.30430903, 33.30430775, 33.30430658, 33.30430528, 33.30430407, 33.30430407, 33.30430269, 33.30430135, 33.30430003, 33.30429869, 33.30429743, 33.30429627, 33.30429513, 33.30429405, 33.30429302, 33.30429204, 33.30429106, 33.30429014, 33.30428918, 33.30428821, 33.30428737, 33.30428647, 33.30428552, 33.30428464, 33.30428368, 33.30428278, 33.30428184, 33.30428095, 33.30428, 33.30427891, 33.30427798, 33.30427698, 33.30427583, 33.30427475, 33.30427366, 33.30427257, 33.30427147, 33.30427032, 33.30426916, 33.30426802, 33.30426685, 33.30426572, 33.30426445, 33.30426329, 33.30426215, 33.30426088, 33.30425969, 33.30425848, 33.30425728, 33.30425617, 33.30425488, 33.30425379, 33.30425252, 33.30425133, 33.30425005, 33.30424881, 33.30424771, 33.3042464, 33.30424517, 33.30424394, 33.30424271, 33.30424152, 33.30424032, 33.30423909, 33.30423791, 33.30423676, 33.30423561, 33.30423456, 33.30423346, 33.30423226, 33.30423114, 33.30422995, 33.30422883, 33.30422763, 33.30422655, 33.3042254, 33.30422436, 33.30422317, 33.30422204, 33.30422098, 33.30421986, 33.30421859, 33.30421756, 33.30421641, 33.30421523, 33.30421412, 33.304213, 33.30421188, 33.30421074, 33.30420964, 33.30420848, 33.30420738, 33.30420621, 33.30420507, 33.30420395, 33.30420281, 33.30420153, 33.30420052, 33.30419933, 33.30419819, 33.30419702, 33.30419581, 33.30419457, 33.30419338, 33.30419214, 33.30419095, 33.30418974, 33.30418852, 33.30418734, 33.30418606, 33.30418491, 33.30418369, 33.3041824, 33.30418115, 33.30417988, 33.30417869, 33.30417738, 33.30417618, 33.30417512, 33.30417397, 33.30417287, 33.30417182, 33.30417087, 33.30416994, 33.3041691, 33.30416829, 33.30416747, 33.30416673, 33.30416589, 33.30416503, 33.30416417, 33.30416322, 33.30416216, 33.30416095, 33.30415971, 33.30415845, 33.30415719, 33.30415595, 33.30415455, 33.30415318, 33.30415192, 33.30415047, 33.30414905, 33.30414765, 33.30414621, 33.30414465, 33.30414307, 33.30414146, 33.30413983, 33.30413813, 33.30413643, 33.30413478, 33.30413306, 33.30413131, 33.30412956, 33.3041278, 33.30412605, 33.30412432, 33.30412256, 33.3041208, 33.30411902, 33.30411728, 33.30411554, 33.30411378, 33.30411208, 33.30411036, 33.30410866, 33.30410698, 33.30410535, 33.30410372, 33.30410208, 33.3041004, 33.30409893, 33.30409728, 33.30409564, 33.30409411, 33.30409238, 33.30409083, 33.30408919, 33.30408752, 33.30408579, 33.30408463, 33.30408295, 33.30408123, 33.30407952, 33.30407785, 33.30407608, 33.30407436, 33.30407267, 33.30407097, 33.30406947, 33.3040679, 33.3040663, 33.30406466, 33.30406313, 33.30406183, 33.30406054, 33.30405932, 33.30405816, 33.30405703, 33.30405602, 33.30405517, 33.30405467, 33.3040537, 33.3040528, 33.3040524, 33.30405185, 33.30405133, 33.30405083, 33.30405001, 33.30404917, 33.30404834, 33.30404755, 33.30404678, 33.30404617, 33.3040451, 33.30404427, 33.3040437, 33.30404327, 33.30404269, 33.3040423, 33.30404184, 33.304042, 33.30404195, 33.304042, 33.304042, 33.30404183, 33.30404183, 33.30404207, 33.30404239, 33.30404283, 33.30404317, 33.30404377, 33.30404442, 33.304045, 33.30404533, 33.30404583, 33.3040465, 33.30404726, 33.30404783, 33.30404846, 33.30404926, 33.30404999, 33.30405036, 33.30405112, 33.30405153, 33.30405183, 33.304052, 33.304052, 33.30405183, 33.30405167, 33.3040515, 33.30405117, 33.30405075, 33.30405026, 33.30404967, 33.30404883, 33.30404801, 33.30404694, 33.3040459, 33.30404467, 33.30404334, 33.30404195, 33.30404048, 33.30403893, 33.30403738, 33.30403588, 33.30403435, 33.30403281, 33.30403119, 33.30402962, 33.30402801, 33.30402632, 33.30402463, 33.30402292, 33.30402118, 33.30401944, 33.30401767, 33.3040159, 33.30401413, 33.30401239, 33.30401065, 33.30400895, 33.30400721, 33.30400546, 33.30400381, 33.3040023, 33.30400069, 33.30399913, 33.3039974, 33.30399581, 33.30399409, 33.3039925, 33.3039909, 33.30398913, 33.30398742, 33.30398599, 33.30398426, 33.30398249, 33.30398069, 33.30397899, 33.30397727, 33.30397559, 33.30397394, 33.30397251, 33.30397095, 33.30396971, 33.30396852, 33.30396728, 33.30396633, 33.30396522, 33.30396436, 33.30396343, 33.3039625, 33.30396166, 33.3039607, 33.30395983, 33.30395917, 33.30395857, 33.30395791, 33.30395748, 33.30395713, 33.30395691, 33.30395638, 33.30395615, 33.30395583, 33.30395537, 33.30395517, 33.303955, 33.30395479, 33.3039545, 33.3039545, 33.30395433, 33.30395449, 33.3039545, 33.30395467, 33.30395498, 33.30395517, 33.30395567, 33.303956, 33.3039565, 33.30395707, 33.30395764, 33.30395801, 33.30395885, 33.30395965, 33.3039606, 33.30396152, 33.30396255, 33.30396377, 33.30396516, 33.30396639, 33.30396774, 33.30396894, 33.3039701, 33.30397116, 33.30397211, 33.30397305, 33.3039739, 33.3039745, 33.30397529, 33.3039759, 33.30397652, 33.30397713, 33.30397757, 33.30397816, 33.30397867, 33.3039791, 33.30397968, 33.30398044, 33.30398105, 33.30398183, 33.30398257, 33.30398351, 33.30398444, 33.30398549, 33.30398658, 33.30398782, 33.30398919, 33.30399063, 33.30399212, 33.30399369, 33.30399528, 33.30399702, 33.3039987, 33.30400043, 33.30400218, 33.30400395, 33.3040057, 33.30400745, 33.30400925, 33.30401104, 33.30401281, 33.30401455, 33.30401628, 33.30401802, 33.30401979, 33.30402153, 33.30402328, 33.30402505, 33.30402683, 33.30402862, 33.30403041, 33.30403217, 33.30403395, 33.30403572, 33.30403748, 33.30403921, 33.30404092, 33.30404255, 33.30404408, 33.3040457, 33.30404725, 33.3040488, 33.30405033, 33.30405186, 33.30405334, 33.30405481, 33.30405638, 33.30405796, 33.30405946, 33.30406102, 33.30406263, 33.30406431, 33.30406604, 33.30406763, 33.30406942, 33.30407121, 33.30407296, 33.3040747, 33.3040764, 33.30407807, 33.3040797, 33.3040813, 33.3040829, 33.30408425, 33.30408563, 33.30408714, 33.30408845, 33.30408992, 33.30409134, 33.3040924, 33.30409342, 33.30409464, 33.30409566, 33.3040967, 33.30409745, 33.30409817, 33.30409869, 33.30409917, 33.30409917, 33.304099, 33.30409883, 33.30409867, 33.30409833, 33.304098, 33.3040975, 33.30409725, 33.3040969, 33.3040965, 33.30409617, 33.3040955, 33.304095, 33.30409449, 33.30409369, 33.30409306, 33.30409246, 33.30409169, 33.304091, 33.30409039, 33.30408964, 33.30408894, 33.3040879, 33.30408698, 33.30408609, 33.30408501, 33.30408417, 33.30408299, 33.30408207, 33.30408113, 33.30408011, 33.30407914, 33.30407806, 33.30407703, 33.30407611, 33.30407529, 33.30407472, 33.30407402, 33.30407336, 33.30407299, 33.3040725, 33.30407233, 33.30407238, 33.30407254, 33.30407298, 33.30407362, 33.30407437, 33.30407524, 33.30407621, 33.30407732, 33.30407842, 33.30407964, 33.30408083, 33.30408199, 33.30408313, 33.30408433, 33.30408554, 33.30408674, 33.30408795, 33.30408915, 33.30409035, 33.30409162, 33.30409282, 33.30409406, 33.3040955, 33.30409691, 33.30409843, 33.30409996, 33.30410145, 33.30410302, 33.30410462, 33.30410625, 33.30410785, 33.30410955, 33.30411127, 33.30411299, 33.30411473, 33.3041165, 33.30411826, 33.30412002, 33.3041218, 33.30412359, 33.30412539, 33.30412719, 33.30412898, 33.30413077, 33.30413253, 33.30413431, 33.30413605, 33.30413782, 33.30413955, 33.30414131, 33.30414306, 33.30414477, 33.30414638, 33.30414793, 33.30414969, 33.30415133, 33.3041531, 33.30415478, 33.30415644, 33.30415803, 33.30415973, 33.30416129, 33.30416291, 33.30416462, 33.30416633, 33.304168, 33.30416971, 33.30417146, 33.30417317, 33.30417477, 33.30417655, 33.3041779, 33.30417967, 33.30418145, 33.30418304, 33.3041847, 33.30418622, 33.30418767, 33.30418921, 33.30419068, 33.30419227, 33.3041935, 33.30419503, 33.30419648, 33.30419779, 33.30419913, 33.30420041, 33.30420146, 33.3042027, 33.30420372, 33.30420454, 33.30420533, 33.30420584, 33.30420642, 33.30420683, 33.30420714, 33.30420733, 33.3042075, 33.30420766, 33.30420718, 33.30420712, 33.30420667, 33.30420623, 33.30420586, 33.3042055, 33.30420497, 33.30420459, 33.30420417, 33.30420367, 33.30420313, 33.30420267, 33.30420217, 33.30420167, 33.30420133, 33.30420076, 33.30420033, 33.30419983, 33.30419933, 33.30419882, 33.30419833, 33.30419768, 33.30419719, 33.30419672, 33.30419617, 33.30419572, 33.30419522, 33.3041945, 33.30419416, 33.30419352, 33.304193, 33.30419279, 33.3041925, 33.30419233, 33.30419233, 33.30419233, 33.30419253, 33.30419283, 33.30419322, 33.30419371, 33.30419407, 33.30419475, 33.30419544, 33.30419625, 33.30419702, 33.30419805, 33.30419893, 33.30419998, 33.30420102, 33.30420207, 33.30420327, 33.30420455, 33.30420578, 33.30420717, 33.30420853, 33.3042099, 33.30421136, 33.30421282, 33.30421437, 33.3042159, 33.30421751, 33.30421912, 33.30422079, 33.30422245, 33.30422418, 33.30422586, 33.30422757, 33.30422929, 33.30423105, 33.30423274, 33.30423443, 33.30423617, 33.3042379, 33.30423964, 33.30424139, 33.30424306, 33.30424479, 33.30424652, 33.304248, 33.30424976, 33.30425154, 33.3042533, 33.30425509, 33.30425689, 33.30425867, 33.30426047, 33.30426226, 33.30426403, 33.30426571, 33.30426735, 33.30426908, 33.30427076, 33.30427248, 33.30427415, 33.30427584, 33.30427738, 33.30427906, 33.30428065, 33.30428205, 33.3042837, 33.30428506, 33.30428645, 33.304288, 33.30428946, 33.30429098, 33.3042922, 33.3042936, 33.30429462, 33.30429558, 33.30429638, 33.304297, 33.30429767, 33.30429832, 33.30429893, 33.30429939, 33.30429967, 33.30429983, 33.30429985, 33.30429968, 33.30429967, 33.3042996, 33.3042994, 33.3042995, 33.30429933, 33.30429917, 33.30429894, 33.30429855, 33.30429831, 33.30429783, 33.30429737, 33.30429697, 33.3042965, 33.30429608, 33.3042955, 33.30429506, 33.3042946, 33.30429398, 33.30429343, 33.30429291, 33.30429233, 33.304292, 33.30429138, 33.304291, 33.30429068, 33.30429037, 33.30428989, 33.30428967, 33.3042895, 33.3042895, 33.3042894, 33.30428929, 33.30428919, 33.3042903, 33.30429148, 33.30429252, 33.30429368, 33.30429483, 33.30429598, 33.30429714, 33.30429826, 33.30429944, 33.30430063, 33.30430181, 33.30430287, 33.30430407, 33.3043052, 33.30430642, 33.30430753, 33.30430867, 33.30430985, 33.30431089, 33.3043121, 33.30431337, 33.30431456, 33.30431579, 33.30431698, 33.30431833, 33.30431958, 33.30432092, 33.30432214, 33.30432347, 33.30432474, 33.30432609, 33.30432748, 33.30432867, 33.30433003, 33.30433133, 33.30433263, 33.30433399, 33.30433523, 33.30433657, 33.30433797, 33.30433937, 33.30434067, 33.304342, 33.30434334, 33.30434457, 33.30434591, 33.30434725, 33.30434867, 33.30434997, 33.30435138, 33.30435259, 33.30435392, 33.3043552, 33.30435656, 33.3043579, 33.30435921, 33.3043605, 33.30436182, 33.3043631, 33.30436435, 33.30436565, 33.30436696, 33.30436823, 33.30436946, 33.30437072, 33.30437193, 33.30437319, 33.30437442, 33.30437563, 33.30437672, 33.30437784, 33.30437898, 33.30438002, 33.30438112, 33.3043822, 33.30438318, 33.30438427, 33.30438535, 33.30438643, 33.30438748, 33.30438854, 33.30438969, 33.30439078, 33.30439199, 33.30439309, 33.30439426, 33.30439549, 33.3043967, 33.30439793, 33.30439917, 33.30440042, 33.30440174, 33.30440304, 33.30440434, 33.30440563, 33.30440699, 33.30440833, 33.30440962, 33.30441093, 33.30441225, 33.30441349, 33.30441479, 33.30441613, 33.30441739, 33.30441862, 33.30441985, 33.3044211, 33.30442234, 33.30442362, 33.30442493, 33.3044262, 33.30442739, 33.30442869, 33.30442987, 33.30443116, 33.30443233, 33.30443357, 33.30443475, 33.30443596, 33.30443707, 33.30443833, 33.30443962, 33.30444082, 33.30444186, 33.30444294]
  out "GPS":T1(graph)=[{"y_long_path"=[250243.79385612707], "x_lat_path"=[3688223.5281783747]}, {"y_long_path"=[250243.757], "x_lat_path"=[3688223.39]}, {"y_long_path"=array[944 elements], "x_lat_path"=array[944 elements]}, {"y_long_path"=[250246.8301, 250246.6716, 250246.4873, 250246.296, 250246.122, 250245.9257, 250245.7732, 250245.5875, 250245.3989, 250245.2166, 250245.0276, 250244.8653, 250244.6749, 250244.5098, 250244.319, 250244.1293, 250243.9404, 250243.757, 250243.5653, 250243.3909, 250243.2171, 250243.0265, 250242.8469, 250242.6561, 250242.4779, 250242.2931, 250242.1112, 250241.9363, 250241.7611, 250241.5908], "x_lat_path"=[3688223.612, 3688223.681, 3688223.731, 3688223.77, 3688223.796, 3688223.82, 3688223.842, 3688223.793, 3688223.791, 3688223.745, 3688223.702, 3688223.665, 3688223.63, 3688223.575, 3688223.538, 3688223.496, 3688223.445, 3688223.39, 3688223.345, 3688223.293, 3688223.242, 3688223.21, 3688223.151, 3688223.108, 3688223.058, 3688223.007, 3688222.954, 3688222.905, 3688222.836, 3688222.787]}]
  out "CTE":dbl=-0.11220359033506931
  in  "K_GPS":dbl=1.0 format="%#_13g"
  out "Tracking_Err(m)":dbl=4862130.802033398
  out "RDDF_Velocity":dbl=126.317125
  in  "Ld(m)":dbl=5.0 format="%#_13g"
  out "GPS_Steer_CMD(Deg)":dbl=2.9943056426975447
  in  "Steer Selector":enum32{"Stanley Method", "Pure Pursuit"}(radio)
  out "xi":dbl=250243.3909
  out "yi":dbl=3688223.293
  out "True_Heading(deg)":dbl format="%#_15g"
  out "UTM X(E) INS":dbl format="%#_13g"
  out "UTM Y(N) INS":dbl format="%#_13g"
  out "GPS_Speed(kph)":dbl format="%#_g kph"
  out "GPS Buffer Read":string
  out "Latitude(deg)":dbl
  out "Logitude(deg)":dbl
  out "Altitude(m)":dbl
  in  "COM7":refnum<visa-resource-name>="COM3" caption="GPS_Com."
  out "CV Loop Time":u32=19558436
  out "Lane_Steer":dbl=3.1742774367668782
  in  "K_Vision":dbl=1.0
  in  "v(Velocity)m/s":dbl=1.0
  out "inference time":string="Total: 586.3ms"
  in  "Binary_image":refnum<k24>(container)
  in  "Current_image":refnum<k24>(container)
  in  "min_area":u32=4
  in  "min_span":u32=4
  in  "max_rmse":u32=1000
  in  "kernel_size":u32=2
  in  "File Path":path=path "C:/Users/JungiHong/OneDrive/Hongik/HI-RACE/2026-01/platform_1_5/ExperimentModules/LaneTracking/forTrainImages/frame_014.jpg"
  in  "UseVideo":bool
  out "Image_String":string
  in  "Image Quality":u32=500
  in  "Cam No.":T2="cam3"
  out "Img_to_Str_Err":errorcluster
  in  "HENES":refnum<visa-resource-name>="COM7"
  out "E-STOP":bool
  out "Remote_M/A":bool
  out "Steer_Feed":dbl=-0.22
  out "Alive_PCU":u8(slide)=29 scale=0.0..254.0
  out "Gear_Feed":u8=1
  out "Speed_Feed(RPM)":dbl format="%#_g rpm"
  out "HENES Buffer Read":string
  out "Speed_Feed(m/s)":dbl
  in  "HLV_A/M":bool=TRUE
  in  "HLV_E-stop":bool
  out "HENES Buffer Write":string
  in  "Input_Spd(cmd)":dbl
  in  "GoBack":bool
  in  "InputSteer(cmd)":dbl
  in  "HLV_Gear":u8=2
  out "PointCloud":T3(graph)=[{"appended array"=[700.0, 700.0, 3500.0, 3500.0, -3500.0, -3500.0, -700.0, -700.0, 700.0], "appended array"=[800.0, -800.0, -800.0, 5200.0, 5200.0, -800.0, -800.0, 800.0, 800.0]}, {"appended array"=[-560.0], "appended array"=[0.0]}, {"appended array"=[-450.0, -450.0, -800.0, -800.0, 0.0, 0.0, -450.0], "appended array"=[100.0, -300.0, -300.0, 1200.0, 1200.0, 100.0, 100.0]}, {"appended array"=[], "appended array"=[]}, {"appended array"=[450.0, 450.0, 800.0, 800.0, 0.0, 0.0, 450.0], "appended array"=[100.0, -300.0, -300.0, 1200.0, 1200.0, 100.0, 100.0]}, {"appended array"=[-1100.0, -1100.0, -1120.0, -1120.0, -1140.0, -1140.0, -1140.0, -1160.0, -1160.0, -1160.0, -1180.0, -1180.0, -1180.0, -1200.0, -1200.0, -1200.0, -1220.0, -1220.0, -1220.0, -1220.0, -1240.0, -1260.0, -1260.0, -1260.0, -1280.0, -1280.0, -1280.0, -1280.0, -1300.0, -1300.0, -1300.0, -1320.0, -1320.0, -1320.0, -1340.0, -1340.0, -1340.0, -1360.0, -1360.0, -1360.0, -1380.0, -1380.0, -1380.0, -1400.0, -1400.0, -1400.0, -1420.0, -1420.0, -1420.0, -1440.0, -1440.0, -1440.0, -1460.0, -1460.0, -1460.0, -1480.0, -1480.0, -1480.0, -1500.0, -1500.0, -1500.0, -1500.0, -1520.0, -1520.0, -1520.0, -1540.0, -1540.0, -1540.0, -1560.0, -1560.0, -1560.0, -1580.0, -1580.0, -1580.0, -1600.0, -1600.0, -1600.0, -1620.0, -1620.0, -1620.0, -1640.0, -1640.0, -1660.0, -1660.0, -1680.0, -1680.0, -1680.0, -1700.0, -1700.0, -1720.0, -1720.0, -1720.0, -1740.0, -1740.0, -1760.0, -1760.0, -1760.0, -1780.0, -1780.0, -1800.0, -1800.0, -1820.0, -1820.0, -1840.0, -1840.0, -1860.0, -1860.0, -1880.0, -1880.0, -1900.0, -1920.0, -1920.0, -1940.0, -1960.0, -1980.0, -2000.0, -2020.0, -2040.0, -2040.0, -2060.0, -2060.0, -2100.0, -2120.0, -2120.0, -2120.0, -2140.0, -2160.0, -2180.0, -2200.0, -2220.0, -2240.0, -2260.0, -2280.0, -2300.0, -2320.0, -2360.0, -2380.0, -2400.0, -2440.0, -2460.0, -2480.0, -2520.0, -2520.0, -2540.0, -2980.0, -2960.0, -2960.0, -2940.0, 1180.0, 1200.0, 1220.0, 1220.0, 1240.0, 1260.0, 1260.0, 1280.0, 1380.0, 1380.0, 1380.0, 1400.0, 1400.0, 1420.0, 1420.0, 1440.0, 1460.0, 3460.0, 3460.0, 3460.0, 3460.0, 3480.0, 3480.0, 3500.0, -1646.388888888889, -2960.0, 1232.5, 1408.888888888889, 3471.4285714285716, 1252.0987654320988, 1271.6975308641975, 1291.2962962962963, 1310.8950617283951, 1330.4938271604938, 1350.0925925925926, 1369.6913580246915, 1389.29012345679], "appended array"=[40.0, 60.0, 60.0, 80.0, 80.0, 100.0, 120.0, 120.0, 140.0, 160.0, 180.0, 200.0, 220.0, 220.0, 240.0, 260.0, 260.0, 280.0, 300.0, 320.0, 340.0, 360.0, 380.0, 400.0, 400.0, 420.0, 440.0, 460.0, 460.0, 480.0, 500.0, 520.0, 540.0, 560.0, 560.0, 580.0, 600.0, 620.0, 640.0, 660.0, 660.0, 680.0, 700.0, 700.0, 720.0, 740.0, 740.0, 760.0, 780.0, 780.0, 800.0, 820.0, 840.0, 860.0, 880.0, 880.0, 900.0, 920.0, 920.0, 940.0, 960.0, 980.0, 980.0, 1000.0, 1020.0, 1020.0, 1040.0, 1060.0, 1080.0, 1100.0, 1120.0, 1120.0, 1140.0, 1160.0, 1160.0, 1180.0, 1200.0, 1220.0, 1240.0, 1260.0, 1280.0, 1300.0, 1320.0, 1340.0, 1360.0, 1380.0, 1400.0, 1420.0, 1440.0, 1460.0, 1480.0, 1500.0, 1520.0, 1540.0, 1560.0, 1580.0, 1600.0, 1620.0, 1640.0, 1660.0, 1680.0, 1700.0, 1720.0, 1740.0, 1780.0, 1800.0, 1820.0, 1840.0, 1860.0, 1920.0, 1940.0, 1980.0, 2020.0, 2080.0, 2120.0, 2160.0, 2180.0, 2220.0, 2240.0, 2280.0, 2320.0, 2360.0, 2400.0, 2420.0, 2460.0, 2500.0, 2540.0, 2580.0, 2620.0, 2680.0, 2720.0, 2780.0, 2820.0, 2880.0, 2920.0, 2980.0, 3020.0, 3080.0, 3160.0, 3220.0, 3280.0, 3340.0, 3380.0, 3440.0, 4340.0, 4360.0, 4380.0, 4420.0, 2560.0, 2580.0, 2560.0, 2540.0, 2540.0, 2540.0, 2520.0, 2520.0, 1720.0, 1700.0, 1680.0, 1680.0, 1660.0, 1660.0, 1640.0, 1660.0, 1660.0, 1800.0, 1780.0, 1760.0, 1740.0, 1720.0, 1700.0, 1700.0, 1304.1666666666667, 4375.0, 2545.0, 1673.3333333333333, 1742.857142857143, 2448.1481481481483, 2351.296296296296, 2254.4444444444443, 2157.5925925925926, 2060.740740740741, 1963.888888888889, 1867.037037037037, 1770.1851851851852]}, {"appended array"=[4.2861222383783204e-13, 0.0], "appended array"=[7000.0, 0.0]}, {"appended array"=[450.0, 450.0, -450.0, -450.0, 450.0], "appended array"=[100.0, 950.0, 950.0, 100.0, 100.0]}]
  in  "격자크기":dbl=20.0
  out "LidarLoop":u32=100
  in  "Ratio_Threshold":i32=4
  in  "min_samples":i32=2
  in  "eps":i32=100
  in  "Spacing":i32=100
  in  "Threshold":i32=2000
  in  "Looking Y":i32=5200
  in  "Looking X":i32=3500
  out "Anthena_Steer":i32
  out "NearSteer":dbl=71.42857142857143
  out "TooClose":bool=TRUE
  out "Clustering Loop":u32=100
  in  "LiDAR":refnum<visa-resource-name>="COM3"
  out "VEstop":bool
  in  "length":dbl=1300.0
  out "LiDAR Buffer Read":string
  out "Clustering Error":errorcluster
  out "GobackROI":cluster{i32[], i32[]}={[450, 450, -450, -450, 450], [100, 950, 950, 100, 100]}
  in  "Stop":bool
  out "TargetDerection":cluster{dbl[], dbl[]}={[4.2861222383783204e-13, 0.0], [7000.0, 0.0]}
  out "Y_arraysREAL":i32[](array[numeric])=[-120, -120, -120, -120, -140, -140, -80, -60, -60]
  out "X_arraysREAL":i32[](array[numeric])=[260, 240, 200, 220, 220, 240, 100, 80, 60]
  out "LookingAt":cluster{i32[], i32[]}={[700, 700, 3500, 3500, -3500, -3500, -700, -700, 700], [800, -800, -800, 5200, 5200, -800, -800, 800, 800]}
  out "NearCarPointsRight":cluster{"ROI_IN_X":dbl[], "ROI_IN_Y":dbl[]}
  out "NearCarROIRight":cluster{i32[], i32[]}={[450, 450, 800, 800, 0, 0, 450], [100, -300, -300, 1200, 1200, 100, 100]}
  out "Clustered":T4={"appended array"=[-1100.0, -1100.0, -1120.0, -1120.0, -1140.0, -1140.0, -1140.0, -1160.0, -1160.0, -1160.0, -1180.0, -1180.0, -1180.0, -1200.0, -1200.0, -1200.0, -1220.0, -1220.0, -1220.0, -1220.0, -1240.0, -1260.0, -1260.0, -1260.0, -1280.0, -1280.0, -1280.0, -1300.0, -1300.0, -1300.0, -1320.0, -1320.0, -1320.0, -1340.0, -1340.0, -1340.0, -1360.0, -1360.0, -1360.0, -1380.0, -1380.0, -1380.0, -1400.0, -1400.0, -1400.0, -1420.0, -1420.0, -1440.0, -1440.0, -1460.0, -1460.0, -1460.0, -1480.0, -1480.0, -1480.0, -1480.0, -1500.0, -1500.0, -1500.0, -1520.0, -1520.0, -1520.0, -1540.0, -1540.0, -1540.0, -1560.0, -1560.0, -1560.0, -1580.0, -1580.0, -1600.0, -1600.0, -1620.0, -1620.0, -1620.0, -1640.0, -1640.0, -1640.0, -1660.0, -1660.0, -1680.0, -1680.0, -1680.0, -1700.0, -1700.0, -1700.0, -1720.0, -1720.0, -1740.0, -1740.0, -1760.0, -1760.0, -1780.0, -1780.0, -1780.0, -1800.0, -1820.0, -1820.0, -1820.0, -1840.0, -1840.0, -1860.0, -1860.0, -1880.0, -1880.0, -1900.0, -1900.0, -1920.0, -1940.0, -1960.0, -1960.0, -1980.0, -2000.0, -2000.0, -2040.0, -2060.0, -2060.0, -2080.0, -2120.0, -2120.0, -2140.0, -2140.0, -2160.0, -2180.0, -2200.0, -2220.0, -2220.0, -2260.0, -2280.0, -2300.0, -2320.0, -2340.0, -2360.0, -2380.0, -2400.0, -2420.0, -2460.0, -2500.0, -2520.0, -2540.0, -2580.0, -2980.0, -2980.0, -2960.0, -2940.0, -2960.0, 1180.0, 1200.0, 1220.0, 1220.0, 1240.0, 1260.0, 1260.0, 1280.0, 1380.0, 1380.0, 1380.0, 1400.0, 1400.0, 1420.0, 1420.0, 1440.0, 1460.0, 3460.0, 3460.0, 3460.0, 3460.0, 3460.0, 3480.0, 3480.0, 3500.0, -1657.163120567376, -2964.0, 1232.5, 1408.888888888889, 3470.0, 1252.0987654320988, 1271.6975308641975, 1291.2962962962963, 1310.8950617283951, 1330.4938271604938, 1350.0925925925926, 1369.6913580246915, 1389.29012345679], "appended array"=[40.0, 60.0, 60.0, 80.0, 80.0, 100.0, 120.0, 120.0, 140.0, 160.0, 180.0, 200.0, 220.0, 220.0, 240.0, 260.0, 260.0, 280.0, 300.0, 320.0, 340.0, 360.0, 380.0, 400.0, 420.0, 440.0, 460.0, 460.0, 480.0, 500.0, 520.0, 540.0, 560.0, 560.0, 580.0, 600.0, 620.0, 640.0, 660.0, 660.0, 680.0, 700.0, 700.0, 720.0, 740.0, 760.0, 780.0, 800.0, 820.0, 840.0, 860.0, 880.0, 880.0, 900.0, 920.0, 940.0, 940.0, 960.0, 980.0, 980.0, 1000.0, 1020.0, 1020.0, 1040.0, 1060.0, 1080.0, 1100.0, 1120.0, 1140.0, 1160.0, 1180.0, 1200.0, 1220.0, 1240.0, 1260.0, 1260.0, 1280.0, 1300.0, 1320.0, 1340.0, 1360.0, 1380.0, 1400.0, 1420.0, 1440.0, 1460.0, 1480.0, 1500.0, 1520.0, 1540.0, 1560.0, 1580.0, 1600.0, 1620.0, 1640.0, 1660.0, 1700.0, 1720.0, 1740.0, 1760.0, 1780.0, 1800.0, 1820.0, 1860.0, 1880.0, 1900.0, 1940.0, 1960.0, 2000.0, 2040.0, 2080.0, 2120.0, 2140.0, 2160.0, 2240.0, 2260.0, 2300.0, 2340.0, 2400.0, 2420.0, 2460.0, 2480.0, 2520.0, 2560.0, 2600.0, 2660.0, 2700.0, 2740.0, 2800.0, 2840.0, 2880.0, 2940.0, 3000.0, 3060.0, 3100.0, 3160.0, 3240.0, 3300.0, 3360.0, 3420.0, 3500.0, 4340.0, 4360.0, 4380.0, 4380.0, 4460.0, 2560.0, 2580.0, 2560.0, 2540.0, 2540.0, 2540.0, 2520.0, 2520.0, 1720.0, 1700.0, 1680.0, 1680.0, 1660.0, 1660.0, 1640.0, 1660.0, 1660.0, 1800.0, 1780.0, 1760.0, 1740.0, 1720.0, 1720.0, 1700.0, 1700.0, 1330.354609929078, 4384.0, 2545.0, 1673.3333333333333, 1740.0, 2448.1481481481483, 2351.296296296296, 2254.4444444444443, 2157.5925925925926, 2060.740740740741, 1963.888888888889, 1867.037037037037, 1770.1851851851852]}
  out "NearCarROILeft":cluster{i32[], i32[]}={[-450, -450, -800, -800, 0, 0, -450], [100, -300, -300, 1200, 1200, 100, 100]}
  out "NearCarPointsLeft":cluster{"ROI_IN_X":dbl[], "ROI_IN_Y":dbl[]}={"ROI_IN_X"=[-560.0], "ROI_IN_Y"=[0.0]}
  out "Y_arrays":dbl[](array[numeric])=[40.0, 60.0, 60.0, 80.0, 80.0, 100.0, 120.0, 120.0, 140.0, 160.0, 180.0, 200.0, 220.0, 220.0, 240.0, 260.0, 260.0, 280.0, 300.0, 320.0, 340.0, 360.0, 380.0, 400.0, 420.0, 440.0, 460.0, 460.0, 480.0, 500.0, 520.0, 540.0, 560.0, 560.0, 580.0, 600.0, 620.0, 640.0, 660.0, 660.0, 680.0, 700.0, 700.0, 720.0, 740.0, 760.0, 780.0, 800.0, 820.0, 840.0, 860.0, 880.0, 880.0, 900.0, 920.0, 940.0, 940.0, 960.0, 980.0, 980.0, 1000.0, 1020.0, 1020.0, 1040.0, 1060.0, 1080.0, 1100.0, 1120.0, 1140.0, 1160.0, 1180.0, 1200.0, 1220.0, 1240.0, 1260.0, 1260.0, 1280.0, 1300.0, 1320.0, 1340.0, 1360.0, 1380.0, 1400.0, 1420.0, 1440.0, 1460.0, 1480.0, 1500.0, 1520.0, 1540.0, 1560.0, 1580.0, 1600.0, 1620.0, 1640.0, 1660.0, 1700.0, 1720.0, 1740.0, 1760.0, 1780.0, 1800.0, 1820.0, 1860.0, 1880.0, 1900.0, 1940.0, 1960.0, 2000.0, 2040.0, 2080.0, 2120.0, 2140.0, 2160.0, 2240.0, 2260.0, 2300.0, 2340.0, 2400.0, 2420.0, 2460.0, 2480.0, 2520.0, 2560.0, 2600.0, 2660.0, 2700.0, 2740.0, 2800.0, 2840.0, 2880.0, 2940.0, 3000.0, 3060.0, 3100.0, 3160.0, 3240.0, 3300.0, 3360.0, 3420.0, 3500.0, 4340.0, 4360.0, 4380.0, 4380.0, 4460.0, 2560.0, 2580.0, 2560.0, 2540.0, 2540.0, 2540.0, 2520.0, 2520.0, 1720.0, 1700.0, 1680.0, 1680.0, 1660.0, 1660.0, 1640.0, 1660.0, 1660.0, 1800.0, 1780.0, 1760.0, 1740.0, 1720.0, 1720.0, 1700.0, 1700.0, 1330.354609929078, 4384.0, 2545.0, 1673.3333333333333, 1740.0, 2448.1481481481483, 2351.296296296296, 2254.4444444444443, 2157.5925925925926, 2060.740740740741, 1963.888888888889, 1867.037037037037, 1770.1851851851852]
  out "X_arrays":dbl[](array[numeric])=[-1100.0, -1100.0, -1120.0, -1120.0, -1140.0, -1140.0, -1140.0, -1160.0, -1160.0, -1160.0, -1180.0, -1180.0, -1180.0, -1200.0, -1200.0, -1200.0, -1220.0, -1220.0, -1220.0, -1220.0, -1240.0, -1260.0, -1260.0, -1260.0, -1280.0, -1280.0, -1280.0, -1300.0, -1300.0, -1300.0, -1320.0, -1320.0, -1320.0, -1340.0, -1340.0, -1340.0, -1360.0, -1360.0, -1360.0, -1380.0, -1380.0, -1380.0, -1400.0, -1400.0, -1400.0, -1420.0, -1420.0, -1440.0, -1440.0, -1460.0, -1460.0, -1460.0, -1480.0, -1480.0, -1480.0, -1480.0, -1500.0, -1500.0, -1500.0, -1520.0, -1520.0, -1520.0, -1540.0, -1540.0, -1540.0, -1560.0, -1560.0, -1560.0, -1580.0, -1580.0, -1600.0, -1600.0, -1620.0, -1620.0, -1620.0, -1640.0, -1640.0, -1640.0, -1660.0, -1660.0, -1680.0, -1680.0, -1680.0, -1700.0, -1700.0, -1700.0, -1720.0, -1720.0, -1740.0, -1740.0, -1760.0, -1760.0, -1780.0, -1780.0, -1780.0, -1800.0, -1820.0, -1820.0, -1820.0, -1840.0, -1840.0, -1860.0, -1860.0, -1880.0, -1880.0, -1900.0, -1900.0, -1920.0, -1940.0, -1960.0, -1960.0, -1980.0, -2000.0, -2000.0, -2040.0, -2060.0, -2060.0, -2080.0, -2120.0, -2120.0, -2140.0, -2140.0, -2160.0, -2180.0, -2200.0, -2220.0, -2220.0, -2260.0, -2280.0, -2300.0, -2320.0, -2340.0, -2360.0, -2380.0, -2400.0, -2420.0, -2460.0, -2500.0, -2520.0, -2540.0, -2580.0, -2980.0, -2980.0, -2960.0, -2940.0, -2960.0, 1180.0, 1200.0, 1220.0, 1220.0, 1240.0, 1260.0, 1260.0, 1280.0, 1380.0, 1380.0, 1380.0, 1400.0, 1400.0, 1420.0, 1420.0, 1440.0, 1460.0, 3460.0, 3460.0, 3460.0, 3460.0, 3460.0, 3480.0, 3480.0, 3500.0, -1657.163120567376, -2964.0, 1232.5, 1408.888888888889, 3470.0, 1252.0987654320988, 1271.6975308641975, 1291.2962962962963, 1310.8950617283951, 1330.4938271604938, 1350.0925925925926, 1369.6913580246915, 1389.29012345679]
types:
  T1 = cluster{"y_long_path":dbl[], "x_lat_path":dbl[]}[]
  T2 = typedef "IMAQdx.ctl" = refnum<k21>
  T3 = cluster{"appended array":dbl[], "appended array":dbl[]}[]
  T4 = cluster{"appended array":dbl[], "appended array":dbl[]}
  T5 = cluster{"HENES_M/A":u8, "HENES_E-Stop":u8, "HENES_Gear":u8, "HENES_Speed":i16, "HENES_Steer":i16, "HENES_Alive":u8}
  T6 = typedef "VISA Flush IO Buffer Mask.ctl" = u16
  T7 = typedef "VISA Set IO Buffer Mask.ctl" = u16
  T8 = cluster{"HLV_M/A_Status":u8, "HLV_E-Stop":u8, "HLV_Gear":u8, "HLV_Speed":i16, "HLV_Steer":i16, "HLV_Alive":u8}
  T9 = cluster{"oldest read timestamp":dbl, "latitude (deg)":dbl, "longitude (deg)":dbl, "ground speed (kph)":dbl, "true track angle (deg)":dbl, "altitude above mean sea level (m)":dbl}
  T10 = cluster{"X_lat_path_Full":dbl[], "Y_long_path_Full":dbl[]}
  T11 = cluster{"Path_lat_arr":dbl[], "Path_long_arr":dbl[]}
  T12 = cluster{"Path_lat_arr":dbl[], "Path_long_arr":dbl[]}[]
  T13 = typedef "IMAQ Image.ctl" = refnum<image>
  T14 = cluster{"Global Rectangle":i32[], "Contours":cluster{"ID":enum32{"External", "Internal"}, "Type":u32, "Coordinates":i32[]}[]}
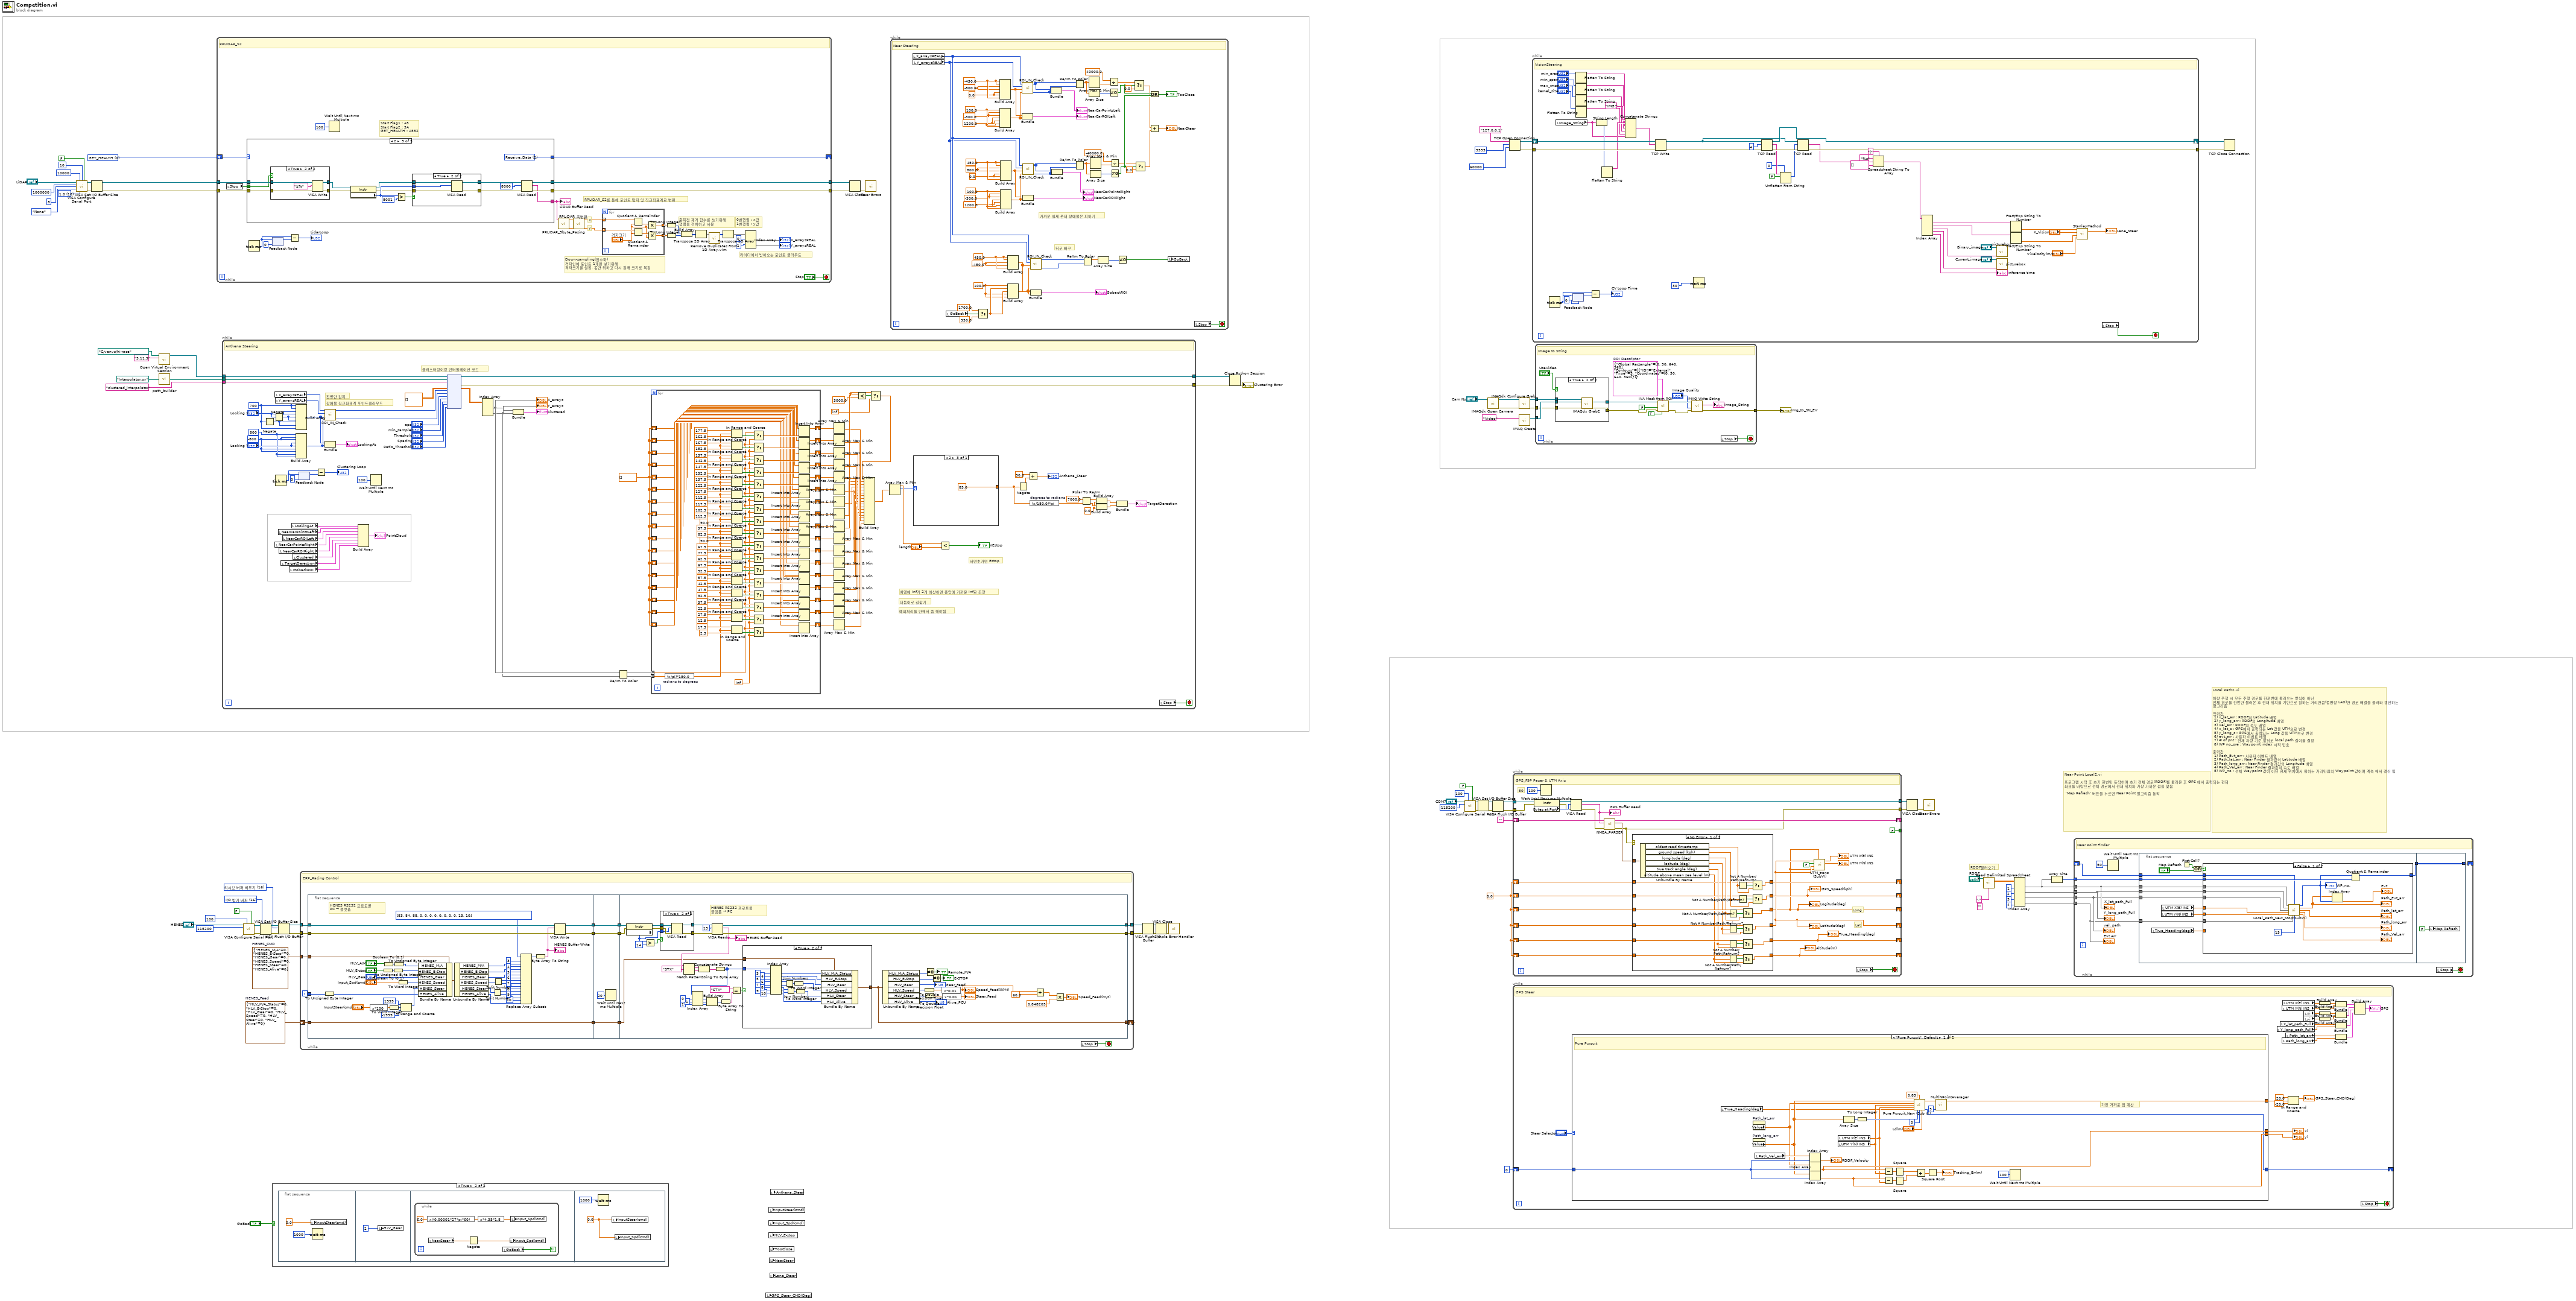
[diagram p0: block diagram]
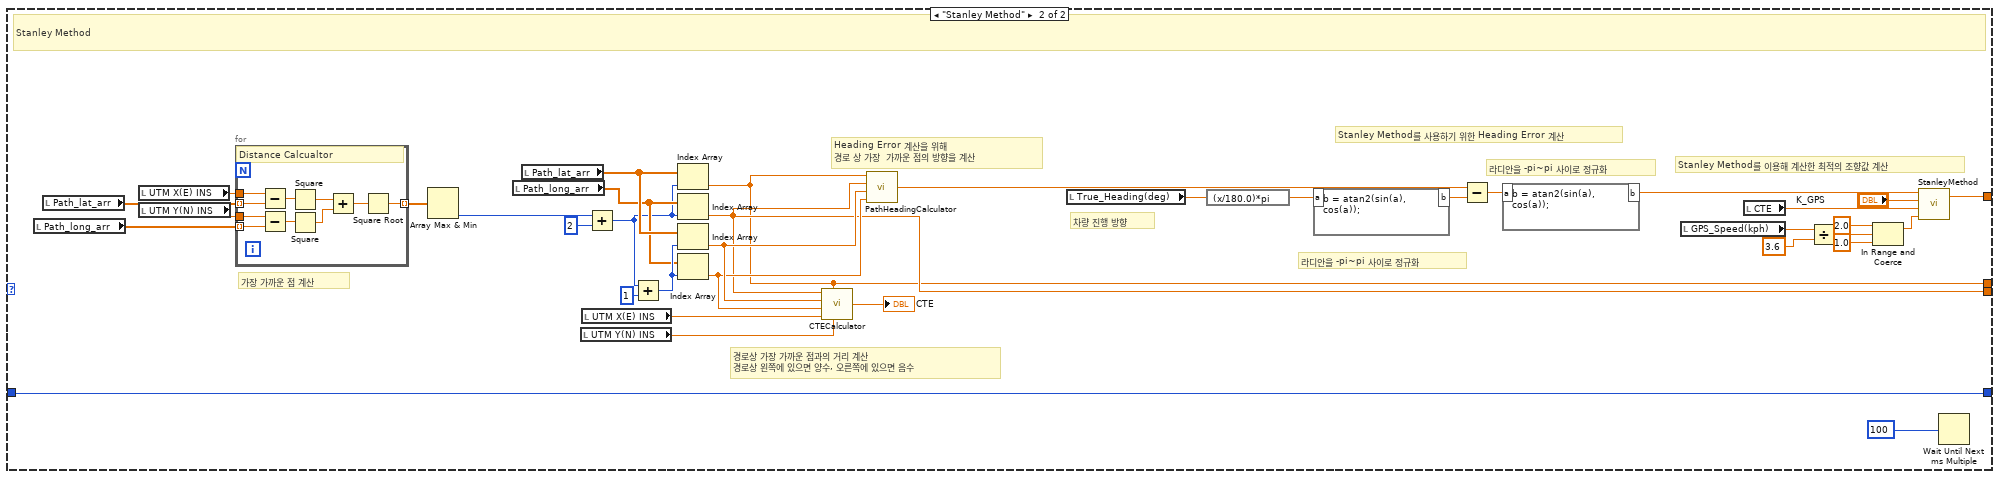
[diagram p4: hidden frame]
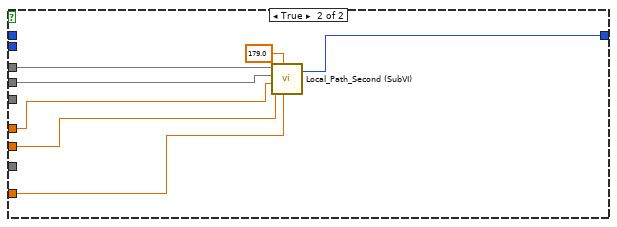
[diagram p5: hidden frame]
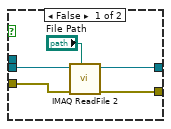
[diagram p6: hidden frame]
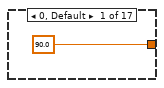
[diagram p9: hidden frame]
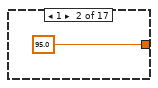
[diagram p10: hidden frame]
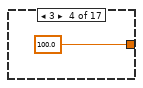
[diagram p11: hidden frame]
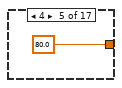
[diagram p12: hidden frame]
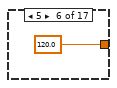
[diagram p13: hidden frame]
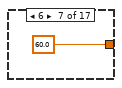
[diagram p14: hidden frame]
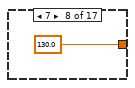
[diagram p15: hidden frame]
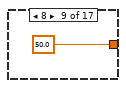
[diagram p16: hidden frame]
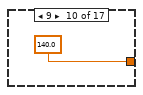
[diagram p17: hidden frame]
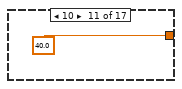
[diagram p18: hidden frame]
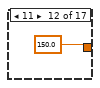
[diagram p19: hidden frame]
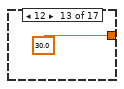
[diagram p20: hidden frame]
diagram:
  w15 = 0.0 ("x")
  (unwired) "" ("delimiter (\\t)")
  w46 = T5 {"HENES_M/A"=0, "HENES_E-Stop"=0, "HENES_Gear"=0, "HENES_Speed"=0, "HENES_Steer"=0, "HENES_Alive"=0}  # HENES_CMD
  w49 = T6 16 items=["리시브 버퍼 비우기"=16, "전달 버퍼 디바이스에 쓰기"=32, "리시브 버퍼 비우기(I/O 없음)"=64, "전달 버퍼 비우기"=128] ("Mask")
  w52 = T7 16 items=["I/O 받기 버퍼"=16, "I/O 전달 버퍼"=32, "I/O 받기와 전달 버퍼"=48] ("Mask")
  w56 = T8 {"HLV_M/A_Status"=0, "HLV_E-Stop"=0, "HLV_Gear"=0, "HLV_Speed"=0, "HLV_Steer"=0, "HLV_Alive"=0}  # HENES_Feed
  w74 = u16 10 items=["1.0"=10, "1.5"=15, "2.0"=20] ("stop bits (10: 1 bit)")
  w76 = u16 0 items=["GET_HEALTH", "SCAN_START", "Receive_Data"]
  # "Near Point Local2.vi\n\n프로그램 시작 후 초기 한번만 동작하며 초기 전체 경로(RDDF)를 불러온 후 GPS 에서 출력되는 현재 좌표를 바탕으로 전체 경로에서 현재 위치와 가장 가까운 점을 찾음\n\n 'Map Refresh' 버튼을 누르면 Near Point 알고리즘 동작"
  # "Local Path2.vi\n\n차량 주행 시 모든 주행 경로를 한꺼번에 불러오는 방식이 아닌\n전체 경로를 한번만 불러온 후 현재 위치를 기반으로 원하는 거리만큼(종뱡항 LAD)만 경로 배열을 불러와 갱신하는 알고리즘\n\n입력값 \n 1) x_lat_arr : RDDF의 Latitude 배열\n 2) y_long_arr : RDDF의 Longitude 배열\n 3) vel_arr : RDDF의 속도 배열\n 4) x_lat_c : GPS에서 출력되는 Lat 값을 UTM으로 변경\n 5) y_long_c : GPS에서 출력되는 Long 값을 UTM으로 변경\n 6) evt_arr : 사용자 이벤트 배열\n 7) # of pnt : 현재 차량 기준 앞뒤로 local path 길이를 결정\n 8) WP no_pre : Waypoint index 시작 번호\n\n출력값 \n 1) Path_Evt_arr : 사용자 이벤트 배열\n 2) Path_lat_arr : Near Finder 결과값의 Latitude 배열\n 3) Path_long_arr : Near Finder 결과값의 Longitude 배열\n 4) Path_Vel_arr : Near Finder 결과값의 속도 배열\n 5) WP_no : 전체 Waypoint 값이 아닌 현재 위치에서 원하는 거리만큼의 Waypoint 값이며 계속 해서 갱신 됨"
  # "RDDF불러오기"
  n1 = call-poly "VISA Configure Serial Port"("VISA resource name"="LiDAR", "timeout (10sec)"=u32 10000, "termination char\n(0xA = '\\n' = LF)"=u8 10 ("termination char\n(0xA = '\\n' = LF)"), "Enable Termination\nChar (T)"=FALSE ("Enable Termination\nChar (T)"), "baud rate (9600)"=u32 1000000, "data bits (8)"=u16 8, "parity (0:none)"=enum16{"None", "Odd", "Even", "Mark", "Space"}."None", "stop bits (10: 1 bit)"=w74) -> ("VISA resource name out"=w83:refnum<visa-resource-name>, "error out"=w82:errorcluster)  [unwired: 6 in]
  n2 = VISA Set I/O Buffer Size(VISA resource name=w83, error in (no error)=w82) -> (VISA resource name out=w78:refnum<visa-resource-name>, error out=w77:errorcluster)  [unwired: 2 in]
  n3 = call-poly <vilib>:"Open Virtual Environment Session.vi"("Python version"="3.11.9", "Env path"=path "C:/venvs/hi-race" ("Name")) -> ("session out"=w65:refnum<k35>)  [unwired: 8 in, 1 out]
  n4 = call "path_builder.vi"("Name"=path "Interpolator.py") -> ("appended path"=w69:path)
  n5 = while {
    tunnel: [w108] -> w87
    tunnel: [w109] -> w86
    tunnel: w78 -> [w117]
    tunnel: w77 -> [w116]
    shift-right: [w115] -> _
    shift-left: w76 -> [w118]
    stop <- "Stop" stop-if-true
    # "라이다에서 받아오는 포인트 클라우드"
    # "RPLIDAR_S2를 통해 포인트 탐지 및 직교좌표계로 변환"
    # "Start Flag1 : A5\nStart Flag2 : 5A \nGET_HEALTH : A552"
    # "0번행렬 : x값\n1번행렬 : y값"
    # "중복점 제거 함수를 쓰기위해\n행렬을 전치하고 사용"
    # "Down-sampling(정수화)\n격자안에 포인트 1개만 넣기위해\n격자크기를 설정, 몫만 취하고 다시 원래 크기로 복원"
    # "Y"
    # "X"
    # "RPLIDAR_S2"
    n6 = local read "Stop"() -> (w114:bool)
    n7 = case shown="2" w118 {
      tunnel: w117 -> [w143 w161 w184]
      tunnel: w116 -> [w142 w160 w183]
      tunnel: [w144 w157 w170] -> w115
      tunnel: [w133 w158 w186] -> w109
      tunnel: [w132 w159 w185] -> w108
      tunnel: w114 -> [_ _ w182]
      tunnel: ["" ("read buffer") w155 w181] -> w93
      frame 0, Default {
        w126 = u16 0 items=["GET_HEALTH", "SCAN_START", "Receive_Data"]
        w127 = u16 1 items=["GET_HEALTH", "SCAN_START", "Receive_Data"]
        n8 = VISA Write(VISA resource name=w143, write buffer="¥R", error in (no error)=w142) -> (VISA resource name out=w137:refnum<visa-resource-name>, error out=w136:errorcluster)  [unwired: 1 out]
        n9 = flat-sequence {
          tunnel: w137 -> [w146]
          tunnel: w136 -> [w145]
          tunnel: [w146] -> w135
          tunnel: [w145] -> w134
          frame #0 {
            n10 = Wait (ms)(milliseconds to wait=u32 5 ("대기 시간 (ms)")) -> ()  [unwired: 1 out]
          }
        }
        n11 = property class="Instr"(reference=w135, error in=w134) -> (reference out=w140:refnum<visa-resource-name>, error out=w139:errorcluster, "Serial Settings:Number of Bytes at Serial Port"=w138:u32)
        n12 = VISA Read(VISA resource name=w140, byte count=w138, error in (no error)=w139) -> (VISA resource name out=w132:refnum<visa-resource-name>, read buffer=w129:string, error out=w133:errorcluster)  [unwired: 1 out]
        n13 = Equal?(x=w129, y="¥Z\u0003\u0000\u0000\u0000\u0006\u0000\u0000\u0000") -> (x = y?=w130:bool)
        n14 = Select(t=w127, s=w130, f=w126) -> (s? t:f=w144:u16)
      }
      frame 1 {
        w148 = u16 2 items=["GET_HEALTH", "SCAN_START", "Receive_Data"]
        w149 = u16 1 items=["GET_HEALTH", "SCAN_START", "Receive_Data"]
        w162 = "¥Z\u0005\u0000\u0000@"
        n15 = VISA Write(VISA resource name=w161, write buffer="¥ \u0000", error in (no error)=w160) -> (VISA resource name out=w164:refnum<visa-resource-name>, error out=w165:errorcluster)  [unwired: 1 out]
        n16 = flat-sequence {
          tunnel: w164 -> [w168]
          tunnel: w165 -> [w167]
          tunnel: [w168] -> w151
          tunnel: [w167] -> w150
          frame #0 {
            n17 = Wait (ms)(milliseconds to wait=u32 5 ("대기 시간 (ms)")) -> ()  [unwired: 1 out]
          }
        }
        n18 = property class="Instr"(reference=w151, error in=w150) -> (reference out=w154:refnum<visa-resource-name>, error out=w153:errorcluster, "Serial Settings:Number of Bytes at Serial Port"=w152:u32)
        n19 = VISA Read(VISA resource name=w154, byte count=w152, error in (no error)=w153) -> (VISA resource name out=w159:refnum<visa-resource-name>, read buffer=w155:string, error out=w158:errorcluster)  [unwired: 1 out]
        n20 = Match Pattern(string=w155, regular expression=w162) -> (match substring=w156:string)  [unwired: 1 in, 3 out]
        n21 = Equal?(x=w156, y=w162) -> (x = y?=w166:bool)
        n22 = Select(t=w148, s=w166, f=w149) -> (s? t:f=w157:u16)
      }
      frame 2 {
        w170 = u16 2 items=["GET_HEALTH", "SCAN_START", "Receive_Data"]
        n23 = case shown="True" w182 {
          tunnel: w184 -> [w195 w199]
          tunnel: w183 -> [w194 w198]
          tunnel: [w195 w197] -> w180
          tunnel: [w194 w196] -> w179
          frame False {
          }
          frame True {
            n24 = VISA Write(VISA resource name=w199, write buffer="¥%", error in (no error)=w198) -> (VISA resource name out=w197:refnum<visa-resource-name>, error out=w196:errorcluster)  [unwired: 1 out]
          }
        }
        n25 = property class="Instr"(reference=w180, error in=w179) -> (reference out=w175:refnum<visa-resource-name>, error out=w174:errorcluster, "Serial Settings:Number of Bytes at Serial Port"=w176:u32)
        n26 = Greater?(x=w176, y=u32 8001) -> (0:w178:bool)
        n27 = case shown="True" w178 {
          tunnel: w175 -> [w188 w193]
          tunnel: w176 -> [_ w192]
          tunnel: w174 -> [w187 w191]
          tunnel: [w188 w190] -> w173
          tunnel: [w187 w189] -> w172
          frame False {
          }
          frame True {
            n28 = VISA Read(VISA resource name=w193, byte count=w192, error in (no error)=w191) -> (VISA resource name out=w190:refnum<visa-resource-name>, error out=w189:errorcluster)  [unwired: 2 out]
          }
        }
        n29 = VISA Read(VISA resource name=w173, byte count=u32 8000, error in (no error)=w172) -> (VISA resource name out=w185:refnum<visa-resource-name>, read buffer=w181:string, error out=w186:errorcluster)  [unwired: 1 out]
      }
    }
    "LiDAR Buffer Read" <- w93
    n30 = Tick Count (ms)() -> (millisecond timer value=w113:u32)
    n31 = feedback #1(u32 0 ("millisecond timer value")) -> (w112:u32)
    n32 = feedback-in #1(w113) -> ()
    n33 = Subtract(x=w113, y=w112) -> (x-y=→"LidarLoop":u32)
    n34 = Wait Until Next ms Multiple(millisecond multiple=u32 100) -> ()  [unwired: 1 out]
    n35 = call "PRLIDAR_5byte_Pasing.vi"("RPLIDAR_Data"=w93) -> ("Theta(deg)"=w96:dbl[], "Distance(mm)"=w97:dbl[])  [unwired: 9 in]
    n36 = call "RPLiDAR_축변환.vi"("Theta(deg)"=w96, "Distance(mm)"=w97) -> ("Y"=w94:dbl[], "X"=w95:dbl[])  [unwired: 8 in]
    n37 = for {
      tunnel: w95 -> [w125] mode=indexing
      tunnel: w94 -> [w124] mode=indexing
      tunnel: [w121] -> w106 mode=indexing
      tunnel: [w120] -> w107 mode=indexing
      n38 = Quotient & Remainder(x=w125, y="격자크기") -> (floor(x/y)=w123:dbl)  [unwired: 1 out]
      n39 = Quotient & Remainder(x=w124, y="격자크기") -> (floor(x/y)=w122:dbl)  [unwired: 1 out]
      n40 = Multiply(x=w123, y="격자크기") -> (x*y=w121:dbl)
      n41 = Multiply(x=w122, y="격자크기") -> (x*y=w120:dbl)
    }
    n42 = To Long Integer(number=w106) -> (32bit integer=w101:i32[])
    n43 = To Long Integer(number=w107) -> (32bit integer=w100:i32[])
    n44 = Build Array(w101, w100) -> (w102:i32[][])
    n45 = Transpose 2D Array(2D array=w102) -> (transposed array=w98:i32[][])
    n46 = call "Remove Duplicates From 1D Array.vim"("array"=w98) -> ("array with duplicates removed"=w99:i32[][])  [unwired: 10 in]
    n47 = Transpose 2D Array(2D array=w99) -> (transposed array=w103:i32[][])
    n48 = Index Array(array=w103, index (row) #1=0 ("index (row)"), index (row) #2=1 ("index (row)")) -> (element #1=→"X_arraysREAL":i32[], element #2=→"Y_arraysREAL":i32[])  [unwired: 2 in]
  }
  n49 = while {
    tunnel: [w302] -> w73
    tunnel: "clustered_interpolator" ("function name") -> [w300]
    tunnel: w69 -> [w299]
    tunnel: w65 -> [w298]
    tunnel: [w301] -> w72
    stop <- w210 stop-if-true
    w213 = dbl[] []
    w215 = 0.0 ("r")
    w275 = -800
    w276 = 800
    w277 = 700
    # "사면초가면 Estop"
    # "배열에 inf가 2개 이상이면 중앙에 가까운 inf로 조향"
    # "예외처리를 안해서 좀 해야됨"
    # "더듬이로 길찾기"
    # "전방만 감지"
    # "장애물 직교좌표계 포인트클라우드"
    # "클러스터링이랑 인터폴레이션 코드"
    # "Anthena Steering"
    n50 = Negate(x=w277) -> (-x=w280:i32)
    n51 = Negate(x="Looking X") -> (-x=w281:i32)
    n52 = local read "X_arraysREAL"() -> (w274:i32[])
    n53 = local read "NearCarPointsRight"() -> (w207:cluster{"ROI_IN_X":dbl[], "ROI_IN_Y":dbl[]})
    n54 = local read "Y_arraysREAL"() -> (w273:i32[])
    n55 = Tick Count (ms)() -> (millisecond timer value=w285:u32)
    n56 = local read "NearCarPointsLeft"() -> (w204:cluster{"ROI_IN_X":dbl[], "ROI_IN_Y":dbl[]})
    n57 = local read "NearCarROIRight"() -> (w208:cluster{i32[], i32[]})
    n58 = local read "TargetDerection"() -> (w202:cluster{dbl[], dbl[]})
    n59 = local read "NearCarROILeft"() -> (w205:cluster{i32[], i32[]})
    n60 = local read "GobackROI"() -> (w201:cluster{i32[], i32[]})
    n61 = local read "LookingAt"() -> (w203:cluster{i32[], i32[]})
    n62 = local read "Clustered"() -> (w209:T4)
    n63 = Build Array(w277, w277, "Looking X", "Looking X", w281, w281, w280, w280, w277) -> (w283:i32[])
    n64 = Build Array(w276, w275, w275, "Looking Y", "Looking Y", w275, w275, w276, w276) -> (w282:i32[])
    n65 = feedback #2(u32 0 ("millisecond timer value")) -> (w286:u32)
    n66 = feedback-in #2(w285) -> ()
    n67 = Subtract(x=w285, y=w286) -> (x-y=→"Clustering Loop":u32)
    n68 = call "ROI_IN_Check.vi"("도형Y좌표"=w282, "도형X좌표"=w283, "LiDAR_Y"=w273, "LiDAR_X"=w274) -> ("ROI_IN_Y"=w271:i32[], "ROI_IN_X"=w272:i32[])  [unwired: 6 in]
    n69 = Bundle(w283, w282) -> (→"LookingAt":cluster{i32[], i32[]})  [unwired: 1 in]
    n70 = Build Array(w203, w204, w205, w207, w208, w209, w202, w201) -> (→"PointCloud":T3)
    n71 = Wait Until Next ms Multiple(millisecond multiple=u32 100) -> ()  [unwired: 1 out]
    n72 = node(w298, w299, w300, dbl[][] [] ("appended array"), w272, w271, "eps", "min_samples", "Threshold", "Spacing", "Ratio_Threshold") -> (w301:refnum<k35>, w302:errorcluster, w297:dbl[][])  [unwired: 8 in, 2 out]
    n73 = Index Array(array=w297) -> (element #1=w212:dbl[], element #2=w211:dbl[])  [unwired: 4 in]
    "X_arrays" <- w212
    "Y_arrays" <- w211
    n74 = Bundle("appended array"=w212, "appended array"=w211) -> (→"Clustered":T4)  [unwired: 1 in]
    n75 = Re/Im To Polar(2:w211, 3:w212) -> (0:w219:dbl[], 1:w220:dbl[])
    n76 = for {
      tunnel: w219 -> [w425] mode=indexing
      tunnel: w220 -> [w347] mode=indexing
      shift-right: [w392] -> w221
      shift-left: w213 -> [w324]
      shift-right: [w391] -> w222
      shift-left: w213 -> [w325]
      shift-right: [w390] -> w223
      shift-left: w213 -> [w326]
      shift-right: [w389] -> w224
      shift-left: w213 -> [w327]
      shift-right: [w388] -> w225
      shift-left: w213 -> [w328]
      shift-right: [w387] -> w226
      shift-left: w213 -> [w329]
      shift-right: [w386] -> w227
      shift-left: w213 -> [w330]
      shift-right: [w385] -> w228
      shift-left: w213 -> [w331]
      shift-right: [w381] -> w234
      shift-left: w213 -> [w332]
      shift-right: [w345] -> w249
      shift-left: w213 -> [w333]
      shift-right: [w344] -> w250
      shift-left: w213 -> [w334]
      shift-right: [w343] -> w251
      shift-left: w213 -> [w335]
      shift-right: [w342] -> w252
      shift-left: w213 -> [w336]
      shift-right: [w338] -> w256
      shift-left: w213 -> [w320]
      shift-right: [w339] -> w255
      shift-left: w213 -> [w321]
      shift-right: [w340] -> w254
      shift-left: w213 -> [w322]
      shift-right: [w341] -> w253
      shift-left: w213 -> [w323]
      w346 = inf
      n77 = expression code="(x/pi)*180.0" "radians to degrees"(w425) -> (w365:dbl)
      n78 = In Range and Coerce(upper limit=177.5, x=w365, lower limit=162.5) -> (In Range?=w352:bool)  [unwired: 1 out]
      n79 = In Range and Coerce(upper limit=167.5, x=w365, lower limit=152.5 ("upper limit")) -> (In Range?=w353:bool)  [unwired: 1 out]
      n80 = In Range and Coerce(upper limit=157.5 ("lower limit"), x=w365, lower limit=142.5 ("upper limit")) -> (In Range?=w354:bool)  [unwired: 1 out]
      n81 = In Range and Coerce(upper limit=147.5 ("lower limit"), x=w365, lower limit=132.5 ("upper limit")) -> (In Range?=w355:bool)  [unwired: 1 out]
      n82 = In Range and Coerce(upper limit=137.5, x=w365, lower limit=122.5) -> (In Range?=w406:bool)  [unwired: 1 out]
      n83 = In Range and Coerce(upper limit=127.5, x=w365, lower limit=112.5) -> (In Range?=w408:bool)  [unwired: 1 out]
      n84 = In Range and Coerce(upper limit=117.5, x=w365, lower limit=102.5) -> (In Range?=w404:bool)  [unwired: 1 out]
      n85 = In Range and Coerce(upper limit=112.5, x=w365, lower limit=90.0) -> (In Range?=w403:bool)  [unwired: 1 out]
      n86 = In Range and Coerce(upper limit=97.5, x=w365, lower limit=82.5) -> (In Range?=w402:bool)  [unwired: 1 out]
      n87 = In Range and Coerce(upper limit=90.0, x=w365, lower limit=67.5) -> (In Range?=w401:bool)  [unwired: 1 out]
      n88 = In Range and Coerce(upper limit=77.5, x=w365, lower limit=62.5) -> (In Range?=w400:bool)  [unwired: 1 out]
      n89 = In Range and Coerce(upper limit=67.5, x=w365, lower limit=52.5) -> (In Range?=w399:bool)  [unwired: 1 out]
      n90 = In Range and Coerce(upper limit=57.5, x=w365, lower limit=42.5) -> (In Range?=w384:bool)  [unwired: 1 out]
      n91 = In Range and Coerce(upper limit=47.5, x=w365, lower limit=32.5) -> (In Range?=w363:bool)  [unwired: 1 out]
      n92 = In Range and Coerce(upper limit=37.5, x=w365, lower limit=22.5) -> (In Range?=w362:bool)  [unwired: 1 out]
      n93 = In Range and Coerce(upper limit=27.5, x=w365, lower limit=12.5) -> (In Range?=w361:bool)  [unwired: 1 out]
      n94 = In Range and Coerce(upper limit=17.5, x=w365, lower limit=2.5) -> (In Range?=w360:bool)  [unwired: 1 out]
      n95 = Select(t=w347, s=w352, f=w346) -> (s? t:f=w351:dbl)
      n96 = Select(t=w347, s=w353, f=w346) -> (s? t:f=w350:dbl)
      n97 = Select(t=w347, s=w354, f=w346) -> (s? t:f=w349:dbl)
      n98 = Select(t=w347, s=w355, f=w346) -> (s? t:f=w348:dbl)
      n99 = Select(t=w347, s=w406, f=w346) -> (s? t:f=w405:dbl)
      n100 = Select(t=w347, s=w408, f=w346) -> (s? t:f=w407:dbl)
      n101 = Select(t=w347, s=w404, f=w346) -> (s? t:f=w393:dbl)
      n102 = Select(t=w347, s=w403, f=w346) -> (s? t:f=w394:dbl)
      n103 = Select(t=w347, s=w402, f=w346) -> (s? t:f=w395:dbl)
      n104 = Select(t=w347, s=w401, f=w346) -> (s? t:f=w396:dbl)
      n105 = Select(t=w347, s=w400, f=w346) -> (s? t:f=w397:dbl)
      n106 = Select(t=w347, s=w399, f=w346) -> (s? t:f=w398:dbl)
      n107 = Select(t=w347, s=w384, f=w346) -> (s? t:f=w364:dbl)
      n108 = Select(t=w347, s=w363, f=w346) -> (s? t:f=w359:dbl)
      n109 = Select(t=w347, s=w362, f=w346) -> (s? t:f=w358:dbl)
      n110 = Select(t=w347, s=w361, f=w346) -> (s? t:f=w357:dbl)
      n111 = Select(t=w347, s=w360, f=w346) -> (s? t:f=w356:dbl)
      n112 = Insert Into Array(array=w320, new element=w351) -> (w338:dbl[])  [unwired: 1 in]
      n113 = Insert Into Array(array=w321, new element=w350) -> (w339:dbl[])  [unwired: 1 in]
      n114 = Insert Into Array(array=w322, new element=w349) -> (w340:dbl[])  [unwired: 1 in]
      n115 = Insert Into Array(array=w323, new element=w348) -> (w341:dbl[])  [unwired: 1 in]
      n116 = Insert Into Array(array=w324, new element=w405) -> (w392:dbl[])  [unwired: 1 in]
      n117 = Insert Into Array(array=w325, new element=w407) -> (w391:dbl[])  [unwired: 1 in]
      n118 = Insert Into Array(array=w326, new element=w393) -> (w390:dbl[])  [unwired: 1 in]
      n119 = Insert Into Array(array=w327, new element=w394) -> (w389:dbl[])  [unwired: 1 in]
      n120 = Insert Into Array(array=w328, new element=w395) -> (w388:dbl[])  [unwired: 1 in]
      n121 = Insert Into Array(array=w329, new element=w396) -> (w387:dbl[])  [unwired: 1 in]
      n122 = Insert Into Array(array=w330, new element=w397) -> (w386:dbl[])  [unwired: 1 in]
      n123 = Insert Into Array(array=w331, new element=w398) -> (w385:dbl[])  [unwired: 1 in]
      n124 = Insert Into Array(array=w332, new element=w364) -> (w381:dbl[])  [unwired: 1 in]
      n125 = Insert Into Array(array=w333, new element=w359) -> (w345:dbl[])  [unwired: 1 in]
      n126 = Insert Into Array(array=w334, new element=w358) -> (w344:dbl[])  [unwired: 1 in]
      n127 = Insert Into Array(array=w335, new element=w357) -> (w343:dbl[])  [unwired: 1 in]
      n128 = Insert Into Array(array=w336, new element=w356) -> (w342:dbl[])  [unwired: 1 in]
    }
    n129 = Array Max & Min(array=w256) -> (min value=w263:dbl)  [unwired: 3 out]
    n130 = Array Max & Min(array=w255) -> (min value=w261:dbl)  [unwired: 3 out]
    n131 = Array Max & Min(array=w254) -> (min value=w259:dbl)  [unwired: 3 out]
    n132 = Array Max & Min(array=w253) -> (min value=w257:dbl)  [unwired: 3 out]
    n133 = Array Max & Min(array=w221) -> (min value=w243:dbl)  [unwired: 3 out]
    n134 = Array Max & Min(array=w222) -> (min value=w241:dbl)  [unwired: 3 out]
    n135 = Array Max & Min(array=w223) -> (min value=w239:dbl)  [unwired: 3 out]
    n136 = Array Max & Min(array=w224) -> (min value=w237:dbl)  [unwired: 3 out]
    n137 = Array Max & Min(array=w225) -> (min value=w269:dbl)  [unwired: 3 out]
    n138 = Array Max & Min(array=w226) -> (min value=w238:dbl)  [unwired: 3 out]
    n139 = Array Max & Min(array=w227) -> (min value=w240:dbl)  [unwired: 3 out]
    n140 = Array Max & Min(array=w228) -> (min value=w242:dbl)  [unwired: 3 out]
    n141 = Array Max & Min(array=w234) -> (min value=w244:dbl)  [unwired: 3 out]
    n142 = Array Max & Min(array=w249) -> (min value=w258:dbl)  [unwired: 3 out]
    n143 = Array Max & Min(array=w250) -> (min value=w260:dbl)  [unwired: 3 out]
    n144 = Array Max & Min(array=w251) -> (min value=w262:dbl)  [unwired: 3 out]
    n145 = Array Max & Min(array=w252) -> (min value=w264:dbl)  [unwired: 3 out]
    n146 = Less?(x=w269, y=3000.0) -> (x < y?=w268:bool)
    n147 = Select(t=w269, s=w268, f=inf) -> (s? t:f=w270:dbl)
    n148 = Build Array(w270, w237, w238, w239, w240, w241, w242, w243, w244, w257, w258, w259, w260, w261, w262, w263, w264) -> (w236:dbl[])
    n149 = Array Max & Min(array=w236) -> (max value=w265:dbl, max index (indices)=w245:i32)  [unwired: 2 out]
    n150 = case shown="2" w245 {
      tunnel: [90.0 95.0 85.0 100.0 80.0 120.0 60.0 130.0 50.0 140.0 40.0 150.0 30.0 160.0 20.0 170.0 10.0] -> w246
      frame 0, Default {
      }
      frame 1 {
      }
      frame 2 {
      }
      frame 3 {
      }
      frame 4 {
      }
      frame 5 {
      }
      frame 6 {
      }
      frame 7 {
      }
      frame 8 {
      }
      frame 9 {
      }
      frame 10 {
      }
      frame 11 {
      }
      frame 12 {
      }
      frame 13 {
      }
      frame 14 {
      }
      frame 15 {
      }
      frame 16 {
      }
    }
    n151 = Less?(x=w265, y="length") -> (x < y?=→"VEstop":bool)
    n152 = Negate(x=w246) -> (-x=w247:dbl)
    n153 = Add(x=90.0, y=w247) -> (x+y=→"Anthena_Steer":dbl)
    n154 = expression code="(x/180.0)*pi" "degrees to radians"(w246) -> (w235:dbl)
    n155 = Polar To Re/Im(2:w235, 3:7000.0 ("r")) -> (0:w230:dbl, 1:w229:dbl)
    n156 = Build Array(w229, w215) -> (w231:dbl[])
    n157 = Build Array(w230, w215) -> (w232:dbl[])
    n158 = Bundle(w231, w232) -> (→"TargetDerection":cluster{dbl[], dbl[]})  [unwired: 1 in]
    n159 = local read "Stop"() -> (w210:bool)
  }
  n160 = call-poly "VISA Configure Serial Port"("VISA resource name"="HENES", "timeout (10sec)"=u32 100, "Enable Termination\nChar (T)"=FALSE ("Enable Termination\nChar (T)"), "baud rate (9600)"=u32 115200) -> ("VISA resource name out"=w48:refnum<visa-resource-name>, "error out"=w47:errorcluster)  [unwired: 10 in]
  n161 = VISA Set I/O Buffer Size(VISA resource name=w48, mask (16)=w52, error in (no error)=w47) -> (VISA resource name out=w51:refnum<visa-resource-name>, error out=w50:errorcluster)  [unwired: 1 in]
  n162 = case shown="True" "GoBack" {
    frame False {
    }
    frame True {
      n163 = flat-sequence {
        frame #0 {
          n164 = local write "InputSteer(cmd)"(0.0 ("InputSteer(cmd)")) -> ()
          n165 = Wait (ms)(milliseconds to wait=u32 1000) -> ()  [unwired: 1 out]
        }
        frame #1 {
          n166 = local write "HLV_Gear"(u8 2 ("HLV_Gear")) -> ()
        }
        frame #2 {
          n167 = while {
            stop <- w431 continue-if-true
            n168 = expression code="x/(0.00001*27*pi*60)"(6.0 ("Input_Spd(kph)")) -> (w434:dbl)
            n169 = local read "NearSteer"() -> (w429:dbl)
            n170 = Negate(x=w429) -> (-x=w430:dbl)
            n171 = expression code="x*4.35*1.8"(w434) -> (w432:dbl)
            n172 = local read "GoBack"() -> (w431:bool)
            n173 = local write "Input_Spd(cmd)"(w430) -> ()
            n174 = local write "Input_Spd(cmd)"(w432) -> ()
          }
        }
        frame #3 {
          w436 = 0.0 ("InputSteer(cmd)")
          n175 = Wait (ms)(milliseconds to wait=u32 1000) -> ()  [unwired: 1 out]
          n176 = local write "InputSteer(cmd)"(w436) -> ()
          n177 = local write "Input_Spd(cmd)"(w436) -> ()
        }
      }
    }
  }
  n178 = VISA Flush I/O Buffer(VISA resource name=w51, mask (16)=w49, error in (no error)=w50) -> (VISA resource name out=w61:refnum<visa-resource-name>, error out=w60:errorcluster)
  n179 = while {
    tunnel: w61 -> [w451]
    tunnel: w60 -> [w450]
    tunnel: [w444] -> w59
    tunnel: [w443] -> w58
    shift-right: [w438] -> _
    shift-left: w56 -> [w441]
    tunnel: w46 -> [w439]
    i -> [w445]
    stop <- w437 stop-if-true
    # "ERP_Racing Control"
    n180 = flat-sequence {
      tunnel: [w494] -> w448
      tunnel: [w493] -> w446
      tunnel: w451 -> [w496]
      tunnel: w450 -> [w495]
      tunnel: w445 -> [w492]
      tunnel: [w491] -> w442
      tunnel: w441 -> [w491]
      tunnel: w439 -> [w490]
      tunnel: [w500] -> w449
      tunnel: w448 -> [w500]
      tunnel: [w499] -> w447
      tunnel: w446 -> [w499]
      tunnel: w442 -> [w497]
      tunnel: [w497] -> w440
      tunnel: w449 -> [w528]
      tunnel: w447 -> [w527]
      tunnel: [w545] -> w444
      tunnel: [w544] -> w443
      tunnel: w440 -> [w519]
      tunnel: [w517] -> w438
      frame #0 {
        # "HENES RS232 프로토콜\nPC → 플랫폼"
        n181 = To Unsigned Byte Integer(number=w492) -> (unsigned 8bit integer=w481:u8)
        n182 = expression code="x*100"("InputSteer(cmd)") -> (w457:dbl)
        n183 = Boolean To (0,1)(Boolean="HLV_E-stop") -> (0, 1=w476:i16)
        n184 = Boolean To (0,1)(Boolean="HLV_A/M") -> (0, 1=w477:i16)
        n185 = To Word Integer(number=w457) -> (16bit integer=w460:i16)
        n186 = To Unsigned Byte Integer(number=w476) -> (unsigned 8bit integer=w474:u8)
        n187 = To Unsigned Byte Integer(number=w477) -> (unsigned 8bit integer=w475:u8)
        n188 = To Word Integer(number="Input_Spd(cmd)") -> (16bit integer=w469:i16)
        n189 = In Range and Coerce(upper limit=i16 1999 ("상위 리미트"), x=w460, lower limit=i16 -1999 ("상위 리미트")) -> (coerced(x)=w468:i16)  [unwired: 1 out]
        n190 = Bundle By Name(cluster=w490, "HENES_M/A"=w475, "HENES_E-Stop"=w474, "HENES_Gear"="HLV_Gear", "HENES_Speed"=w469, "HENES_Steer"=w468, "HENES_Alive"=w481) -> (w483:T5)
        n191 = Unbundle By Name(w483) -> ("HENES_M/A"=w471:u8, "HENES_E-Stop"=w470:u8, "HENES_Gear"=w461:u8, "HENES_Speed"=w464:i16, "HENES_Steer"=w467:i16, "HENES_Alive"=w480:u8)
        n192 = Split Number(x=w467) -> (hi(x)=w466:u8, lo(x)=w465:u8)
        n193 = Split Number(x=w464) -> (hi(x)=w463:u8, lo(x)=w462:u8)
        n194 = Replace Array Subset(array=u8[] [83, 84, 88, 0, 0, 0, 0, 0, 0, 0, 0, 13, 10] ("unsigned byte array"), new element #1=w471, index #1=3, new element #2=w470, index #2=4, new element #3=w461, index #3=5, new element #4=w463, index #4=6, new element #5=w462, index #5=7, new element #6=w466, index #6=8, new element #7=w465, index #7=9, new element #8=w480, index #8=10) -> (w455:u8[])
        n195 = Byte Array To String(unsigned byte array=w455) -> (string=w456:string)
        "HENES Buffer Write" <- w456
        n196 = VISA Write(VISA resource name=w496, write buffer=w456, error in (no error)=w495) -> (VISA resource name out=w494:refnum<visa-resource-name>, error out=w493:errorcluster)  [unwired: 1 out]
      }
      frame #1 {
        n197 = Wait Until Next ms Multiple(millisecond multiple=u32 20 ("대기 시간 (ms)")) -> ()  [unwired: 1 out]
      }
      frame #2 {
        # "HENES RS232 프로토콜\n플랫폼 → PC"
        n198 = property class="Instr"(reference=w528, error in=w527) -> (reference out=w508:refnum<visa-resource-name>, error out=w507:errorcluster, "Serial Settings:Number of Bytes at Serial Port"=w506:u32)
        n199 = Greater?(x=w506, y=u32 14) -> (0:w524:bool)
        n200 = case shown="True" w524 {
          tunnel: w508 -> [w572 w577]
          tunnel: w507 -> [w571 w576]
          tunnel: [w572 w575] -> w526
          tunnel: [w571 w574] -> w525
          tunnel: w506 -> [_ w573]
          frame False {
          }
          frame True {
            n201 = VISA Read(VISA resource name=w577, byte count=w573, error in (no error)=w576) -> (VISA resource name out=w575:refnum<visa-resource-name>, error out=w574:errorcluster)  [unwired: 2 out]
          }
        }
        n202 = VISA Read(VISA resource name=w526, byte count=u32 13, error in (no error)=w525) -> (VISA resource name out=w545:refnum<visa-resource-name>, read buffer=w543:string, error out=w544:errorcluster)  [unwired: 1 out]
        "HENES Buffer Read" <- w543
        n203 = Match Pattern(string=w543, regular expression="STX") -> (match substring=w540:string, after substring=w541:string)  [unwired: 1 in, 2 out]
        n204 = Concatenate Strings(w540, w541) -> (w539:string)
        n205 = String To Byte Array(string=w539) -> (unsigned byte array=w521:u8[])
        n206 = Index Array(array=w521, index #1=0, index #2=1, index #3=2) -> (element #1=w534:u8, element #2=w533:u8, element #3=w532:u8)
        n207 = Build Array(w534, w533, w532) -> (w531:u8[])
        n208 = Byte Array To String(unsigned byte array=w531) -> (string=w529:string)
        n209 = Equal?(x="STX", y=w529) -> (x = y?=w520:bool)
        n210 = case shown="True" w520 {
          tunnel: w521 -> [_ w570]
          tunnel: [w547 w557] -> w517
          tunnel: w519 -> [w547 w559]
          frame False {
          }
          frame True {
            n211 = Index Array(array=w570, index #1=3, index #2=4, index #3=5, index #4=6, index #5=7, index #6=8, index #7=9, index #8=10) -> (element #1=w558:u8, element #2=w556:u8, element #3=w555:u8, element #4=w554:u8, element #5=w553:u8, element #6=w551:u8, element #7=w550:u8, element #8=w548:u8)
            n212 = Join Numbers(hi=w554, lo=w553) -> ((hi.lo)=w561:u16)
            n213 = Join Numbers(hi=w551, lo=w550) -> ((hi.lo)=w560:u16)
            n214 = To Word Integer(number=w561) -> (16bit integer=w552:i16)
            n215 = To Word Integer(number=w560) -> (16bit integer=w549:i16)
            n216 = Bundle By Name(cluster=w559, "HLV_M/A_Status"=w558, "HLV_E-Stop"=w556, "HLV_Gear"=w555, "HLV_Speed"=w552, "HLV_Steer"=w549, "HLV_Alive"=w548) -> (w557:T8)
          }
        }
        n217 = Unbundle By Name(w517) -> ("HLV_M/A_Status"=w518:u8, "HLV_E-Stop"=w512:u8, "HLV_Gear"=→"Gear_Feed":u8, "HLV_Speed"=w510:i16, "HLV_Steer"=w509:i16, "HLV_Alive"=→"Alive_PCU":u8)
        n218 = To Double Precision Float(number=w510) -> (double precision float=w522:dbl)
        n219 = To Double Precision Float(number=w509) -> (double precision float=w515:dbl)
        n220 = Not Equal To 0?(x=w518) -> (x != 0?=→"Remote_M/A":bool)
        n221 = Not Equal To 0?(x=w512) -> (x != 0?=→"E-STOP":bool)
        n222 = expression code="x*0.01"(w522) -> (w501:dbl)
        "Speed_Feed(RPM)" <- w501
        n223 = expression code="x*0.01"(w515) -> (→"Steer_Feed":dbl)
        n224 = Divide(x=w501, y=60.0) -> (x/y=w505:dbl)
        n225 = Multiply(x=w505, y=0.848205) -> (x*y=→"Speed_Feed(m/s)":dbl)
      }
    }
    n226 = local read "Stop"() -> (w437:bool)
  }
  n227 = local read "GPS_Steer_CMD(Deg)"() -> ()  [unwired: 1 in]
  n228 = local read "InputSteer(cmd)"() -> ()  [unwired: 1 in]
  n229 = local read "Input_Spd(cmd)"() -> ()  [unwired: 1 in]
  n230 = local read "HLV_E-stop"() -> ()  [unwired: 1 in]
  n231 = local read "TooClose"() -> ()  [unwired: 1 in]
  n232 = local read "NearSteer"() -> ()  [unwired: 1 in]
  n233 = local read "Lane_Steer"() -> ()  [unwired: 1 in]
  n234 = local read "Anthena_Steer"() -> ()  [unwired: 1 in]
  n235 = VISA Close(VISA resource name=w87, error in (no error)=w86) -> (error out=w88:errorcluster)
  n236 = call <vilib>:"Clear Errors.vi"("error in (no error)"=w88) -> ()  [unwired: 5 in, 2 out]
  n237 = while {
    stop <- w579 stop-if-true
    w582 = -450.0 ("element")
    w584 = 100.0 ("element")
    w583 = 450.0 ("element")
    w605 = 1200.0 ("f")
    w599 = 1200.0 ("element")
    w602 = 0.0 ("element")
    w606 = -300.0 ("element")
    w603 = 800.0 ("element")
    w607 = 100.0 ("element")
    w604 = 450.0 ("element")
    w596 = 0.0 ("element")
    w600 = -300.0 ("element")
    w597 = -800.0 ("element")
    w601 = 100.0 ("element")
    w598 = -450.0 ("element")
    # "뒤로 빠꾸"
    # "가까운 실제 존재 장애물은 피하기"
    # "Neer Steering"
    n238 = local read "X_arraysREAL"() -> (w581:i32[])
    n239 = local read "Y_arraysREAL"() -> (w580:i32[])
    n240 = local read "GoBack"() -> (w578:bool)
    n241 = Select(t=1700.0, s=w578, f=950.0 ("element")) -> (s? t:f=w595:dbl)
    n242 = Build Array(w598, w598, w597, w597, w596, w596, w598) -> (w621:dbl[])
    n243 = Build Array(w601, w600, w600, w599, w599, w601, w601) -> (w620:dbl[])
    n244 = Build Array(w604, w604, w603, w603, w602, w602, w604) -> (w613:dbl[])
    n245 = Build Array(w607, w606, w606, w605, w605, w607, w607) -> (w614:dbl[])
    n246 = Build Array(w583, w583, w582, w582, w583) -> (w592:dbl[])
    n247 = Build Array(w584, w595, w595, w584, w584) -> (w591:dbl[])
    n248 = call "ROI_IN_Check.vi"("도형Y좌표"=w620, "도형X좌표"=w621, "LiDAR_Y"=w580, "LiDAR_X"=w581) -> ("ROI_IN_Y"=w623:i32[], "ROI_IN_X"=w622:i32[])  [unwired: 6 in]
    n249 = Bundle(w621, w620) -> (→"NearCarROILeft":cluster{dbl[], dbl[]})  [unwired: 1 in]
    n250 = call "ROI_IN_Check.vi"("도형Y좌표"=w614, "도형X좌표"=w613, "LiDAR_Y"=w580, "LiDAR_X"=w581) -> ("ROI_IN_Y"=w626:i32[], "ROI_IN_X"=w625:i32[])  [unwired: 6 in]
    n251 = Bundle(w613, w614) -> (→"NearCarROIRight":cluster{dbl[], dbl[]})  [unwired: 1 in]
    n252 = call "ROI_IN_Check.vi"("도형Y좌표"=w591, "도형X좌표"=w592, "LiDAR_Y"=w580, "LiDAR_X"=w581) -> ("ROI_IN_Y"=w588:i32[], "ROI_IN_X"=w589:i32[])  [unwired: 6 in]
    n253 = Bundle(w592, w591) -> (→"GobackROI":cluster{dbl[], dbl[]})  [unwired: 1 in]
    n254 = Bundle("ROI_IN_X"=w622, "ROI_IN_Y"=w623) -> (→"NearCarPointsLeft":cluster{"ROI_IN_X":i32[], "ROI_IN_Y":i32[]})  [unwired: 1 in]
    n255 = Bundle("ROI_IN_X"=w625, "ROI_IN_Y"=w626) -> (→"NearCarPointsRight":cluster{"ROI_IN_X":i32[], "ROI_IN_Y":i32[]})  [unwired: 1 in]
    n256 = Re/Im To Polar(2:w623, 3:w622) -> (1:w624:dbl[])  [unwired: 1 out]
    n257 = Re/Im To Polar(2:w626, 3:w625) -> (1:w627:dbl[])  [unwired: 1 out]
    n258 = Re/Im To Polar(2:w588, 3:w589) -> (1:w587:dbl[])  [unwired: 1 out]
    n259 = Array Max & Min(array=w624) -> (min value=w628:dbl)  [unwired: 3 out]
    n260 = Array Size(array=w624) -> (size(s)=w619:i32)
    n261 = Array Max & Min(array=w627) -> (min value=w629:dbl)  [unwired: 3 out]
    n262 = Array Size(array=w627) -> (size(s)=w612:i32)
    n263 = Array Size(array=w587) -> (size(s)=w593:i32)
    n264 = Divide(x=40000.0, y=w628) -> (x/y=w631:dbl)
    n265 = Not Equal To 0?(x=w619) -> (x != 0?=w636:bool)
    n266 = Divide(x=-40000.0, y=w629) -> (x/y=w633:dbl)
    n267 = Not Equal To 0?(x=w612) -> (x != 0?=w635:bool)
    n268 = Not Equal To 0?(x=w593) -> (x != 0?=w594:bool)
    n269 = Select(t=w631, s=w636, f=0.0) -> (s? t:f=w632:dbl)
    n270 = Select(t=w633, s=w635, f=0.0) -> (s? t:f=w634:dbl)
    n271 = Or(x=w636, y=w635) -> (x .or. y?=→"TooClose":bool)
    n272 = Add(x=w632, y=w634) -> (x+y=→"NearSteer":dbl)
    n273 = local write "GoBack"(w594) -> ()
    n274 = local read "Stop"() -> (w579:bool)
  }
  n275 = VISA Flush I/O Buffer(VISA resource name=w59, error in (no error)=w58) -> (VISA resource name out=w62:refnum<visa-resource-name>, error out=w63:errorcluster)  [unwired: 1 in]
  n276 = VISA Close(VISA resource name=w62, error in (no error)=w63) -> (error out=w57:errorcluster)
  n277 = call <vilib>:"Simple Error Handler.vi"("error in (no error)"=w57) -> ()  [unwired: 4 in, 5 out]
  n278 = Close Python Session(session in=w72, error in=w73) -> (11:→"Clustering Error":errorcluster)
  n279 = call-poly "VISA Configure Serial Port"("VISA resource name"="COM7", "timeout (10sec)"=u32 100, "Enable Termination\nChar (T)"=FALSE ("Enable Termination\nChar (T)"), "baud rate (9600)"=u32 115200) -> ("VISA resource name out"=w21:refnum<visa-resource-name>, "error out"=w20:errorcluster)  [unwired: 10 in]
  n280 = VISA Set I/O Buffer Size(VISA resource name=w21, error in (no error)=w20) -> (VISA resource name out=w26:refnum<visa-resource-name>, error out=w25:errorcluster)  [unwired: 2 in]
  n281 = call <vilib>:"IMAQdx Open Camera.vi"("Session In"="Cam No.") -> ("error out"=w34:errorcluster, "Session Out"=w33:T2)  [unwired: 9 in]
  n282 = VISA Flush I/O Buffer(VISA resource name=w26, error in (no error)=w25) -> (VISA resource name out=w24:refnum<visa-resource-name>, error out=w23:errorcluster)  [unwired: 1 in]
  n283 = TCP Open Connection(address="127.0.0.1", remote port or service name=u16 5555, timeout ms (60000)=60000) -> (connection ID=w42:refnum<k5>, error out=w41:errorcluster)  [unwired: 2 in]
  n284 = while {
    tunnel: w24 -> [w665]
    tunnel: w23 -> [w663]
    tunnel: [w667] -> w29
    tunnel: [w655] -> w27
    shift-right: [w656] -> _
    shift-left: "" -> [w660]
    shift-right: [w643] -> _
    shift-left: w15 -> [w654]
    shift-right: [w641] -> _
    shift-left: w15 -> [w653]
    shift-right: [w642] -> _
    shift-left: w15 -> [w652]
    shift-right: [w648] -> _
    shift-left: w15 -> [w651]
    shift-right: [w647] -> _
    shift-left: w15 -> [w650]
    tunnel: [FALSE] -> _
    shift-right: [w639] -> _
    shift-left: w15 -> [w640]
    stop <- w638 stop-if-true
    # "Lat"
    # "Long"
    # "50"
    # "GPS_F9P Paser & UTM Axis"
    n285 = property class="Instr"(reference=w665, error in=w663) -> (reference out=w664:refnum<visa-resource-name>, error out=w662:errorcluster, "Bytes at Port"=w666:u32)
    n286 = Wait Until Next ms Multiple(millisecond multiple=u32 100) -> ()  [unwired: 1 out]
    n287 = VISA Read(VISA resource name=w664, byte count=w666, error in (no error)=w662) -> (VISA resource name out=w667:refnum<visa-resource-name>, read buffer=w659:string, error out=w657:errorcluster)  [unwired: 1 out]
    "GPS Buffer Read" <- w659
    n288 = call "NMEA_PARSER.vi"("previous partial sentence"=w660, "sensor data"=w659, "error in (no error)"=w657) -> ("remaining partial sentence"=w656:string, "GPS data"=w658:T9, "error out"=w655:errorcluster)  [unwired: 5 in]
    n289 = case shown="No Error" w655 {
      tunnel: w658 -> [w692 _]
      tunnel: w653 -> [w688 w698]
      tunnel: w652 -> [w687 w697]
      tunnel: w651 -> [w686 w696]
      tunnel: [w682 w698] -> w641
      tunnel: [w681 w697] -> w642
      tunnel: [w680 w696] -> w648
      tunnel: w654 -> [w677 w695]
      tunnel: [w676 w695] -> w643
      tunnel: w650 -> [w673 w694]
      tunnel: [w672 w694] -> w647
      tunnel: [w669 w693] -> w639
      tunnel: w640 -> [w668 w693]
      frame No Error {
        n290 = Unbundle By Name(w692) -> ("oldest read timestamp"=w674:dbl, "ground speed (kph)"=w678:dbl, "longitude (deg)"=w685:dbl, "latitude (deg)"=w684:dbl, "true track angle (deg)"=w683:dbl, "altitude above mean sea level (m)"=w670:dbl)
        n291 = Not A Number/Path/Refnum?(number/path/refnum=w685) -> (NaN/Path/Refnum?=w691:bool)
        n292 = Not A Number/Path/Refnum?(number/path/refnum=w684) -> (NaN/Path/Refnum?=w690:bool)
        n293 = Not A Number/Path/Refnum?(number/path/refnum=w683) -> (NaN/Path/Refnum?=w689:bool)
        n294 = Not A Number/Path/Refnum?(number/path/refnum=w670) -> (NaN/Path/Refnum?=w671:bool)
        n295 = Not A Number/Path/Refnum?(number/path/refnum=w674) -> (NaN/Path/Refnum?=w675:bool)
        n296 = Not A Number/Path/Refnum?(number/path/refnum=w678) -> (NaN/Path/Refnum?=w679:bool)
        n297 = Select(t=w688, s=w691, f=w685) -> (s? t:f=w682:dbl)
        n298 = Select(t=w687, s=w690, f=w684) -> (s? t:f=w681:dbl)
        n299 = Select(t=w686, s=w689, f=w683) -> (s? t:f=w680:dbl)
        n300 = Select(t=w668, s=w671, f=w670) -> (s? t:f=w669:dbl)
        n301 = Select(t=w673, s=w675, f=w674) -> (s? t:f=w672:dbl)
        n302 = Select(t=w677, s=w679, f=w678) -> (s? t:f=w676:dbl)
      }
      frame Error {
        # "Invalid data points."
      }
    }
    "True_Heading(deg)" <- w648
    "GPS_Speed(kph)" <- w643
    "Latitude(deg)" <- w642
    "Logitude(deg)" <- w641
    "Altitude(m)" <- w639
    n303 = call "UTM_trans (SubVI).vi"("Long_Deg"=w641, "long"=w641, "lat"=w642, "East?West?"=FALSE, "Lat_Deg"=w642) -> ("UTM_Y(Northing)"=→"UTM Y(N) INS":dbl, "UTM_X(Easting)"=→"UTM X(E) INS":dbl)  [unwired: 2 out]
    n304 = local read "Stop"() -> (w638:bool)
  }
  n305 = while {
    shift-right: [w708] -> _
    shift-left: 0 ("Index(near vehicle)") -> [w707]
    stop <- w706 stop-if-true
    # "GPS Steer"
    n306 = case shown="\"Pure Pursuit\", Default" "Steer Selector" {
      tunnel: [w751 w784] -> w702
      tunnel: [w729 w752] -> w708
      tunnel: w707 -> [w734 w752]
      tunnel: [w732 w757] -> w704
      tunnel: [w733 w756] -> w703
      frame "Pure Pursuit", Default {
        # "가장 가까운 점 계산"
        # "Pure Pursuit"
        n307 = local read "True_Heading(deg)"() -> (w726:dbl)
        n308 = property on="Path_lat_arr" class="Arr (strict)"() -> ("Value"=w731:dbl[])  [unwired: 2 in, 2 out]
        n309 = property on="Path_long_arr" class="Arr (strict)"() -> ("Value"=w730:dbl[])  [unwired: 2 in, 2 out]
        n310 = local read "Path_Vel_arr"() -> (w735:dbl[])
        n311 = Index Array(array=w735, index=w734) -> (element=→"RDDF_Velocity":dbl)
        n312 = Index Array(array=w731, index=w734) -> (element=w733:dbl)
        n313 = Index Array(array=w730, index=w734) -> (element=w732:dbl)
        n314 = local read "UTM Y(N) INS"() -> (w728:dbl)
        n315 = local read "UTM X(E) INS"() -> (w727:dbl)
        n316 = Array Size(array=w730) -> (size(s)=w744:i32)
        n317 = To Long Integer(number=w744) -> (32bit integer=w743:i32)
        n318 = Subtract(x=w733, y=w728) -> (x-y=w750:dbl)
        n319 = Subtract(x=w732, y=w727) -> (x-y=w749:dbl)
        n320 = Square(x=w750) -> (x^2=w748:dbl)
        n321 = Square(x=w749) -> (x^2=w747:dbl)
        n322 = call "Pure Pursuit_New (Sub VI).vi"("x_lat_path"=w730, "L"=0.85, "y_long_path"=w731, "X_Current"=w728, "Y_Current"=w727, "Heading_Current"=w726, "#pnt"=w743, "WP no_pre"=0, "LAD"="Ld(m)") -> ("Steer_CMD(Deg)"=w739:dbl, "Index(near vehicle)"=w729:i32)  [unwired: 3 in, 2 out]
        n323 = Add(x=w748, y=w747) -> (x+y=w746:dbl)
        n324 = Square Root(x=w746) -> (sqrt(x)=→"Tracking_Err(m)":dbl)
        n325 = call "MultiNPointAverager.vi"("N point average"=3 ("WP no_pre"), "Data_input"=w739) -> ("숫자형"=w751:dbl)  [unwired: 9 in]
        n326 = Wait Until Next ms Multiple(millisecond multiple=u32 100 ("ms 배수")) -> ()  [unwired: 1 out]
      }
      frame "Stanley Method" {
        # "Stanley Method를 이용해 계산한 최적의 조향값 계산"
        # "차량 진행 방향"
        # "Stanley Method를 사용하기 위한 Heading Error 계산"
        # "라디안을 -pi~pi 사이로 정규화"
        # "라디안을 -pi~pi 사이로 정규화"
        # "경로상 가장 가까운 점과의 거리 계산\n경로상 왼쪽에 있으면 양수, 오른쪽에 있으면 음수"
        # "Heading Error 계산을 위해\n경로 상 가장  가까운 점의 방향을 계산"
        # "가장 가까운 점 계산"
        # "Stanley Method"
        n327 = local read "Path_long_arr"() -> (w782:dbl[])
        n328 = local read "Path_lat_arr"() -> (w781:dbl[])
        n329 = local read "UTM X(E) INS"() -> (w779:dbl)
        n330 = local read "UTM Y(N) INS"() -> (w780:dbl)
        n331 = for {
          tunnel: w779 -> [w797]
          tunnel: w780 -> [w796]
          tunnel: w781 -> [w788] mode=indexing
          tunnel: w782 -> [w789] mode=indexing
          tunnel: [w790] -> w783 mode=indexing
          # "Distance Calcualtor"
          n332 = Subtract(x=w797, y=w788) -> (x-y=w795:dbl)
          n333 = Subtract(x=w796, y=w789) -> (x-y=w794:dbl)
          n334 = Square(x=w795) -> (x^2=w793:dbl)
          n335 = Square(x=w794) -> (x^2=w792:dbl)
          n336 = Add(x=w793, y=w792) -> (x+y=w791:dbl)
          n337 = Square Root(x=w791) -> (sqrt(x)=w790:dbl)
        }
        n338 = Array Max & Min(array=w783) -> (min index (indices)=w754:i32)  [unwired: 3 out]
        n339 = local read "Path_long_arr"() -> (w773:dbl[])
        n340 = local read "Path_lat_arr"() -> (w774:dbl[])
        n341 = local read "UTM Y(N) INS"() -> (w777:dbl)
        n342 = local read "UTM X(E) INS"() -> (w778:dbl)
        n343 = Add(x=w754, y=2) -> (x+y=w753:i32)
        n344 = Add(x=w753, y=1) -> (x+y=w776:i32)
        n345 = Index Array(array=w774, index=w753) -> (element=w756:dbl)
        n346 = Index Array(array=w773, index=w753) -> (element=w757:dbl)
        n347 = Index Array(array=w774, index=w776) -> (element=w772:dbl)
        n348 = Index Array(array=w773, index=w776) -> (element=w771:dbl)
        n349 = call "CTECalculator.vi"("yp"=w777, "xi"=w756, "xp"=w778, "yi1"=w771, "xi1"=w772, "yi"=w757) -> ("CTE"=→"CTE":dbl)
        n350 = call "PathHeadingCalculator.vi"("yi1"=w771, "xi1"=w772, "yi"=w757, "xi"=w756) -> ("PathHeading"=w786:dbl)
        n351 = local read "True_Heading(deg)"() -> (w766:dbl)
        n352 = expression code="(x/180.0)*pi" ("degrees to radians")(w766) -> (w768:dbl)
        n353 = formula code="b = atan2(sin(a), cos(a));"("a"=w768) -> ("b"=w767:dbl)
        n354 = Subtract(x=w786, y=w767) -> (x-y=w769:dbl)
        n355 = formula code="b = atan2(sin(a), cos(a));"("a"=w769) -> ("b"=w785:dbl)
        n356 = local read "GPS_Speed(kph)"() -> (w765:dbl)
        n357 = local read "CTE"() -> (w761:dbl)
        n358 = Divide(x=w765, y=3.6) -> (x/y=w764:dbl)
        n359 = In Range and Coerce(upper limit=2.0, x=w764, lower limit=1.0) -> (coerced(x)=w763:dbl)  [unwired: 1 out]
        n360 = call "StanleyMethod.vi"("v(Velocity)m/s"=w763, "e(Cross-Track Err)m/s"=w761, "k(Gain)"="K_GPS", "ψ(Heading Err)radian"=w785) -> ("δ(OutputSteer)degrees"=w784:dbl)  [unwired: 1 out]
        n361 = Wait Until Next ms Multiple(millisecond multiple=u32 100) -> ()  [unwired: 1 out]
      }
    }
    "xi" <- w703
    "yi" <- w704
    n362 = local read "Y_long_path_Full"() -> (w724:dbl[])
    n363 = local read "X_lat_path_Full"() -> (w725:dbl[])
    n364 = local read "UTM Y(N) INS"() -> (w722:dbl)
    n365 = local read "Path_long_arr"() -> (w718:dbl[])
    n366 = local read "UTM X(E) INS"() -> (w723:dbl)
    n367 = local read "Path_lat_arr"() -> (w719:dbl[])
    n368 = In Range and Coerce(upper limit=20.0, x=w702, lower limit=-20.0) -> (coerced(x)=→"GPS_Steer_CMD(Deg)":dbl)  [unwired: 1 out]
    n369 = local read "xi"() -> (w717:dbl)
    n370 = local read "yi"() -> (w716:dbl)
    n371 = Build Array(w723) -> (w721:dbl[])
    n372 = Build Array(w722) -> (w720:dbl[])
    n373 = Build Array(w717) -> (w715:dbl[])
    n374 = Build Array(w716) -> (w714:dbl[])
    n375 = Bundle(w721, w720) -> (w713:cluster{dbl[], dbl[]})  [unwired: 1 in]
    n376 = Bundle(w715, w714) -> (w712:cluster{dbl[], dbl[]})  [unwired: 1 in]
    n377 = Bundle("X_lat_path_Full"=w725, "Y_long_path_Full"=w724) -> (w711:T10)  [unwired: 1 in]
    n378 = Bundle("Path_lat_arr"=w719, "Path_long_arr"=w718) -> (w710:T11)  [unwired: 1 in]
    n379 = Build Array(w713, w712, w711, w710) -> (→"GPS":T12)
    n380 = local read "Stop"() -> (w706:bool)
  }
  n381 = call <vilib>:"IMAQdx Configure Grab.vi"("error in"=w34, "Session In"=w33) -> ("error out"=w35:errorcluster, "Session Out"=w32:T2)  [unwired: 8 in]
  n382 = call "IMAQ Create"("Image Name"="Video") -> ("New Image"=w31:T13)  [unwired: 4 in, 1 out]
  n383 = while {
    tunnel: w41 -> [w818]
    tunnel: [w830] -> w43
    shift-right: [w828] -> w44
    shift-left: w42 -> [w819]
    stop <- w800 stop-if-true
    # "VisionSteering"
    n384 = Tick Count (ms)() -> (millisecond timer value=w845:u32)
    n385 = local read "Image_String"() -> (w801:string)
    n386 = feedback #3(u32 0 ("millisecond timer value")) -> (w844:u32)
    n387 = feedback-in #3(w845) -> ()
    n388 = Flatten To String(anything="min_area") -> (data string=w805:string)  [unwired: 3 in, 2 out]
    n389 = Flatten To String(anything="min_span") -> (data string=w804:string)  [unwired: 3 in, 2 out]
    n390 = Flatten To String(anything="max_rmse") -> (data string=w803:string)  [unwired: 3 in, 2 out]
    n391 = Flatten To String(anything="kernel_size") -> (data string=w802:string)  [unwired: 3 in, 2 out]
    n392 = Subtract(x=w845, y=w844) -> (x-y=→"CV Loop Time":u32)
    n393 = String Length(string=w801) -> (length=w816:i32)
    n394 = Flatten To String(anything=w816) -> (data string=w815:string)  [unwired: 3 in, 2 out]
    n395 = Concatenate Strings("IMG!" ("Image_String"), w815, w805, w804, w803, w802, w801) -> (w813:string)
    n396 = TCP Write(connection ID=w819, data in=w813, error in (no error)=w818) -> (connection ID out=w820:refnum<k5>, error out=w821:errorcluster)  [unwired: 1 in, 1 out]
    n397 = Wait (ms)(milliseconds to wait=u32 30) -> ()  [unwired: 1 out]
    n398 = TCP Read(connection ID=w820, bytes to read=4, error in (no error)=w821) -> (connection ID out=w828:refnum<k5>, data out=w825:string, error out=w827:errorcluster)  [unwired: 2 in]
    n399 = Unflatten From String(type=u32 0 ("CV Loop Time 2"), binary string=w825, data includes array or string size? (T)=FALSE) -> (value=w826:u32)  [unwired: 2 in, 2 out]
    n400 = TCP Read(connection ID=w820, bytes to read=w826, error in (no error)=w827) -> (data out=w829:string, error out=w830:errorcluster)  [unwired: 2 in, 1 out]
    n401 = Spreadsheet String To Array(delimiter (Tab)="|", format string="%s", spreadsheet string=w829, array type (2D Dbl)=string[] []) -> (array=w831:string[])
    n402 = Index Array(array=w831) -> (element #1=w834:string, element #2=w833:string, element #3=w812:string, element #4=w799:string, element #5=→"inference time":string)  [unwired: 5 in]
    n403 = call "picturebox.vi"("s"=w812, "PictureBox"="Binary_image") -> ()  [unwired: 10 in]
    n404 = call "picturebox.vi"("s"=w799, "PictureBox"="Current_image") -> ()  [unwired: 10 in]
    n405 = Fract/Exp String To Number(string=w834) -> (number=w840:dbl)  [unwired: 3 in, 1 out]
    n406 = Fract/Exp String To Number(string=w833) -> (number=w839:dbl)  [unwired: 3 in, 1 out]
    n407 = call "StanleyMethod.vi"("v(Velocity)m/s"="v(Velocity)m/s", "e(Cross-Track Err)m/s"=w839, "k(Gain)"="K_Vision", "ψ(Heading Err)radian"=w840) -> ("δ(OutputSteer)degrees"=→"Lane_Steer":dbl)  [unwired: 1 out]
    n408 = local read "Stop"() -> (w800:bool)
  }
  n409 = while {
    tunnel: w31 -> [w859]
    tunnel: w32 -> [w858]
    tunnel: w35 -> [w857]
    tunnel: [w849] -> w37
    stop <- w860 stop-if-true
    w854 = T14 {"Global Rectangle"=[0, 50, 640, 360], "Contours"=[{"ID"=enum."External", "Type"=3, "Coordinates"=[0, 50, 640, 360]}]}  # ROI Descriptor
    # "Image to String"
    n410 = case shown="True" "UseVideo" {
      tunnel: w859 -> [w863 w870]
      tunnel: [w865 w869] -> w847
      tunnel: [w864 w868] -> w852
      tunnel: w858 -> [_ w867]
      tunnel: w857 -> [w861 w866]
      frame False {
        n411 = call "IMAQ ReadFile 2"("File Path"="File Path", "error in (no error)"=w861, "Image"=w863) -> ("error out"=w865:errorcluster, "Image Out"=w864:T13)  [unwired: 4 in, 3 out]
      }
      frame True {
        n412 = call <vilib>:"IMAQdx Grab2.vi"("error in"=w866, "Image In"=w870, "Session In"=w867) -> ("error out"=w869:errorcluster, "Image Out"=w868:T13)  [unwired: 5 in, 2 out]
      }
    }
    n413 = call <vilib>:"IVA Mask from ROI.vi"("Shrink"=TRUE, "ROI Descriptor"=w854, "error in (no error)"=w847, "Out / In"=FALSE, "Image Src"=w852) -> ("error out"=w846:errorcluster, "Image Out"=w850:T13)  [unwired: 5 out]
    n414 = call-poly "IMAQ Write String"("error in (no error)"=w846, "Image Quality"="Image Quality", "Image"=w850) -> ("error out"=w849:errorcluster, "FileString"=→"Image_String":string)  [unwired: 6 in, 1 out]
    n415 = local read "Stop"() -> (w860:bool)
  }
  "Img_to_Str_Err" <- w37
  n416 = VISA Close(VISA resource name=w29, error in (no error)=w27) -> (error out=w28:errorcluster)
  n417 = call <vilib>:"Clear Errors.vi"("error in (no error)"=w28) -> ()  [unwired: 5 in, 2 out]
  n418 = call-poly <vilib>:"Read Delimited Spreadsheet.vi"("file path (dialog if empty)"="RDDF", "delimiter (\\t)"="," ("delimiter (\\t)")) -> ("all rows"=w8:dbl[][])  [unwired: 8 in, 5 out]
  n419 = Index Array(array=w8, index (col) #1=1 ("비활성화된 인덱스 (열)"), index (col) #2=2 ("인덱스 (열)"), index (col) #3=3 ("인덱스 (열)"), index (col) #4=4 ("인덱스 (열)")) -> (element #1=w10:dbl[], element #2=w11:dbl[], element #3=w13:dbl[], element #4=w12:dbl[])  [unwired: 4 in]
  n420 = Array Size(array=w10) -> (size(s)=w9:i32)
  n421 = while {
    shift-right: [w879] -> _
    shift-left: _ -> [w880]
    tunnel: w9 -> [w877]
    tunnel: w13 -> [w872]
    tunnel: w11 -> [w874]
    tunnel: w10 -> [w873]
    tunnel: w12 -> [w871]
    stop <- w876 stop-if-true
    # "Near Point Finder"
    n422 = Wait Until Next ms Multiple(millisecond multiple=u32 50) -> ()  [unwired: 1 out]
    n423 = flat-sequence {
      tunnel: [w892] -> w878
      tunnel: w880 -> [w893]
      tunnel: w877 -> [w888]
      tunnel: w872 -> [w887]
      tunnel: w874 -> [w886]
      tunnel: w873 -> [w885]
      tunnel: w871 -> [w884]
      tunnel: [w918] -> w879
      tunnel: w878 -> [w918]
      frame #0 {
        n424 = local read "True_Heading(deg)"() -> (w881:dbl)
        n425 = local read "UTM Y(N) INS"() -> (w882:dbl)
        n426 = local read "UTM X(E) INS"() -> (w883:dbl)
        n427 = First Call?() -> (First Call?: T/F=w890:bool)
        n428 = Or(x=w890, y="Map Refresh") -> (x .or. y?=w891:bool)
        n429 = case shown="False" w891 {
          tunnel: w885 -> [w905 w916]
          tunnel: w886 -> [w906 w915]
          tunnel: w893 -> [w904 _]
          tunnel: w887 -> [w907 _]
          tunnel: w888 -> [w908 _]
          tunnel: [w909 w913] -> w892
          tunnel: w884 -> [w903 _]
          tunnel: w883 -> [w902 w912]
          tunnel: w882 -> [w901 w911]
          tunnel: w881 -> [_ w910]
          frame False {
            n430 = call "Local_Path_New_Stop(SubVI).vi"("x_lat_arr"=w905, "WP no_pre"=w904, "y_long_arr"=w906, "vel_arr"=w907, "x_lat_c"=w902, "y_long_c"=w901, "evt_arr"=w903, "# of pnt"=15) -> ("INDEX(Near Point)"=w900:i32, "Evt(Local)"=w897:dbl[], "Lat(Local)"=→"Path_lat_arr":dbl[], "Long(Local)"=→"Path_long_arr":dbl[], "Vel(Local)"=→"Path_Vel_arr":dbl[])  [unwired: 3 in]
            "WP_no." <- w900
            "Path_Evt_arr" <- w897
            n431 = Index Array(array=w897, index=w900) -> (element=→"Evt":dbl)
            n432 = Quotient & Remainder(x=w900, y=w908) -> (x-y*floor(x/y)=w909:i32)  [unwired: 1 out]
          }
          frame True {
            n433 = call "Local_Path_Second (SubVI).vi"("heading_deg"=w910, "heading_limit"=179.0, "y_long"=w911, "x_lat"=w912, "Y_long_path"=w915, "X_lat_path"=w916) -> ("Index(near vehicle)"=w913:i32)  [unwired: 1 out]
          }
        }
      }
      frame #1 {
        n434 = local write "Map Refresh"(FALSE ("Refresh")) -> ()
      }
    }
    n435 = local read "Stop"() -> (w876:bool)
    "X_lat_path_Full" <- w873
    "vel. path" <- w872
    "Y_long_path_Full" <- w874
    "Evt.Arr" <- w871
  }
  n436 = TCP Close Connection(connection ID=w44, error in (no error)=w43) -> ()  [unwired: 1 in, 2 out]
